vi "Dashboard Main.vi"() -> ()   [LabVIEW 2017]
uses:
  Config Cluster.ctl
  Plate Assignments.ctl
  <vilib>/Utility/miscctls.llb/LVRowAndColumnTypeDef.ctl
  <vilib>/event_ctls.llb/eventvkey.ctl
  <vilib>/Rock Robotics/Network Tables/NT Read Numeric Array.vi
  <vilib>/Rock Robotics/Network Tables/NT Read Boolean.vi
  <vilib>/Utility/file.llb/Read Delimited Spreadsheet (DBL).vi
  <vilib>/Rock Robotics/Network Tables/NT Read Boolean Array.vi
  <vilib>/Rock Robotics/Network Tables/NT Write Boolean Array.vi
  <vilib>/Rock Robotics/Network Tables/NT Write Boolean.vi
  <vilib>/Rock Robotics/Network Tables/NT Write Numeric Array.vi
  <vilib>/Utility/file.llb/Write Delimited Spreadsheet (DBL).vi
  <vilib>/Rock Robotics/WPI/Dashboard/WPI_DashboardLogging Global.vi
  <vilib>/Utility/file.llb/Read Delimited Spreadsheet (string).vi
  <vilib>/Utility/file.llb/Write Delimited Spreadsheet (string).vi
  <vilib>/Rock Robotics/Network Tables/NT Write String Array.vi
panel:
  in  "Camera Settings Right":T1={"Frame Rate"=30, "Compression"=30, "Size"=1, "DB Camera Config"=FALSE} {"Frame Rate" scale=1.0..30.0; "Compression" scale=100.0..-1.0; "Size" items=["640x480", "320x240", "160x120"]}
  in  "Camera Name Right":string(combo)="No Camera Selection"
  out "Camera Info":cluster{"Mbps LED":bool, "Mbps":dbl, "fps":dbl} {"fps" format="%#.1g"; "Mbps" format="%#.1g"}
  in  "Camera Settings":T1={"Frame Rate"=30, "Compression"=30, "Size"=1, "DB Camera Config"=FALSE} {"Frame Rate" scale=1.0..30.0; "Compression" scale=100.0..-1.0; "Size" items=["640x480", "320x240", "160x120"]}
  in  "TCP":refnum<k5>
  in  "Rec Mode":enum32{"Stop", "Record", "Playback"}(radio)
  out "Robot IP":string
  out "Image Message":string="Timeout in Camera Communications"
  in  "Dashboard Tab":T2(tab)=enum."Drive"
  out "Auto Frame":dbl
  out "Gyro":dbl
  out "Current Lift Position 2":dbl
  out "Lift Reference Point 2":dbl
  out "Zero Feedback":bool
  in  "Reset Lift to Start Config":bool
  in  "Zero Gyro":bool
  out "Flush feedback":bool
  in  "Flush Network Table":bool
  in  "Invert Manual Lift":bool
  out "Pause Cycling":bool
  in  "Config Cluster File Path":path=path "C:/Users/PhyXTGears/Desktop/ConfigCSV - 2018.csv"
  in  "Auto Array File Path":path=path "C:/Users/PhyXTGears/Desktop/AutoCSV - 2018.csv"
  out "Alt Numeric Process":dbl
  out "Alt Process Variable":bool
  in  "Select Auto":string(combo)="Select Autonomous ..."
  out "NT Connection":bool
  out "JS1 Z":dbl(slide) scale=-1.0..1.0 scale format="%#_2e"
  out "JS1 Graph":cluster{"X":dbl, "Y":dbl}[](graph)
  out "JS1 Buttons":T3
  out "JS2 Z":dbl(slide) scale=-1.0..1.0 scale format="%#_2e"
  out "JS2 Graph":cluster{"X":dbl, "Y":dbl}[](graph)
  out "JS2 Buttons":T3
  out "Mode":T4(ring)=enum."Auto Disabled"
  out "Camera Image Right":T5(plugin-control)
  out "Plate Assignments":T6
  out "Lift Reference Point":dbl
  out "Ramp Tail Status":bool=TRUE
  out "Intake Short":bool
  out "Intake Long":bool
  out "Drive Orientation":bool
  out "Current Lift Position":dbl
  out "BR Spin":dbl(knob) scale=0.0..360.0
  out "BL Spin":dbl(knob) scale=0.0..360.0
  out "FR Spin":dbl(knob) scale=0.0..360.0
  out "FL Spin":dbl(knob) scale=0.0..360.0
  out "Cube Secured":bool
  out "Cube Seen":bool
  out "Gyro":dbl(knob) scale=-180.0..180.0
  out "Lift Position":dbl(slide) scale=0.0..240000.0
  out "Time Remaining":dbl=135.0 format="%#.0f"
  out "Auto Indicator":string="Error - Driver Station Not Running"
  in  "Auto Select":string(combo)="Drive Forward"
  out "Notify LED":bool
  out "Notify":string="Error - DS Not Running"
  out "Auto Ready":bool
  out "# of Cells\nPresent":dbl
  out "Feedback":bool
  in  "Write to Sheet":bool
  in  "Arm Write":bool
  in  "Arm Read":bool
  in  "Read Sheet":bool
  in  "Auto Array":string[][](array[string])=[["", ""], ["", ""], ["", ""], ["", ""], ["", ""], ["", ""], ["", ""], ["", ""], ["", ""], ["", ""], ["", ""], ["", ""], ["", ""], ["", ""], ["", ""], ["", ""], ["", ""], ["", ""], ["", ""], ["", ""], ["", ""], ["", ""], ["", ""], ["", ""], ["", ""], ["", ""], ["", ""], ["", ""]]
  out "Auto Array 2":string[][](array[string])
  in  "Arm Write Config":bool
  in  "Config Cluster":T7
  in  "Arm Read Config":bool
  in  "Write to Sheet 2":bool
  out "Feedback 2":bool
  in  "Read Sheet 2":bool
  out "Control Feedback":bool
  in  "Zero BR":bool
  in  "Zero BL":bool
  in  "Zero FR":bool
  in  "Zero FL":bool
  out "BL Rverse":bool
  out "FL Rverse":bool
  out "BR Rverse":bool
  out "FR Rverse":bool
  in  "Enable Zero Ctrls":bool
  in  "Read Zeros from File":bool
  in  "Save Zeros to File":bool
  in  "Zero Drive":bool
  out "FR Encoder":dbl
  out "Swerve Zeros":dbl[](array[numeric])
  out "BR Spin":dbl
  out "BL Spin":dbl
  out "FR Spin":dbl
  out "FL Spin":dbl
  out "Spin Wheels":cluster{dbl, dbl, dbl, dbl}(knob) scale=0.0..360.0
  in  "Test Slider":dbl(slide) scale=0.0..100.0 scale format="%#_3g"
  in  "On/Off":bool caption="Solenoid"
  in  "Test Name":u16(ring) items=["Select the test to run..."]
  in  "Test Tree":string(tree)
  in  "Motor":cluster{"Value":dbl, "Enable":bool} {"Value" scale=-1.0..1.0 scale format="%#_3g"}
  out "Progress":T8 {"Test Progress" scale=0.0..100.0}
  in  "Rev/Fwd":cluster{"Forward":bool, "Reverse":bool}
  in  "Test Ring":u16(ring) items=["Monochrome", "Color"]
  out "Cmd Status":string
  in  "Execute Command":bool
  in  "Command Params":string[][](table)
  in  "Command Selection":i32(listbox)
  in  "CheckList":i32(listbox)
  out "Tree":string(tree)
  out "Camera Image":T5(plugin-control)
  out "Background":bool
  in  "Camera Name":string(combo)="No Camera Selection"
  # "HW"
  # "HW"
  # "Joysticks"
  # "Auto Commands Ref\nS - Stop/Abort\nT - Movement Angle\nM - Distance to move\nA -  Angle to face\nL - Lift Position"
  # "Oppo"
  # "Scale"
  # "Ours"
  # "See\nBackend\ntab for \ncmd refs"
  # "Intake"
  # "Servos"
  # "FL-Red\nFR-Orng\nBL-Grn\nBR-Blu"
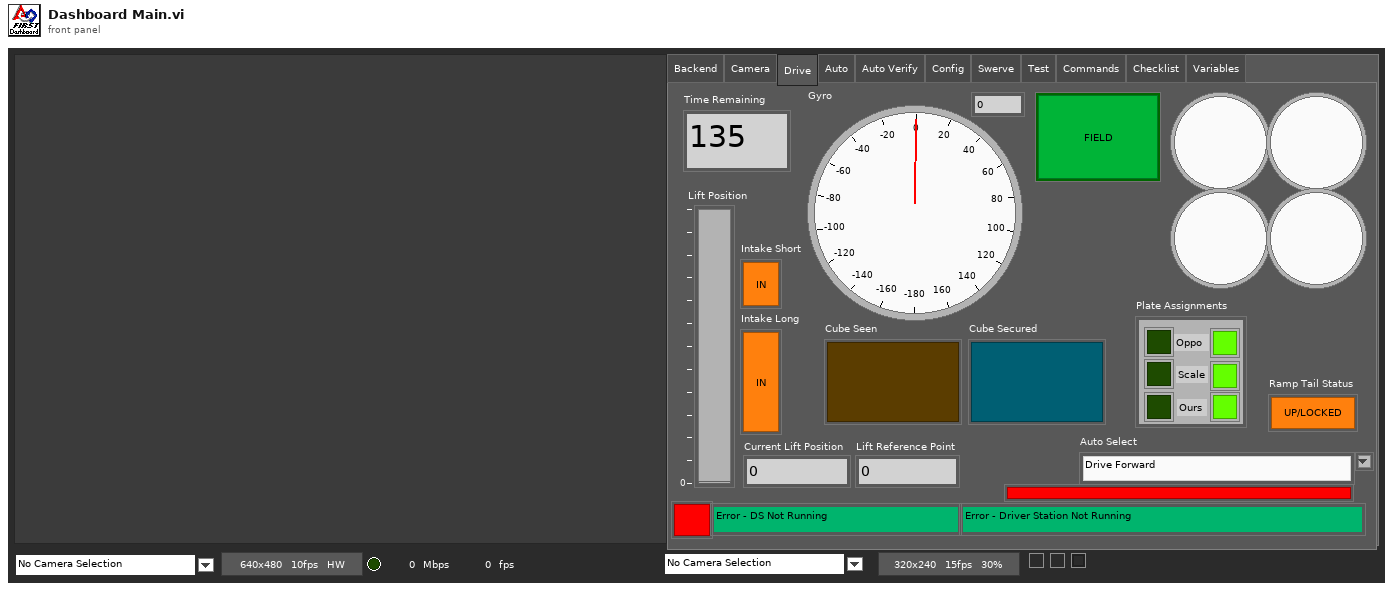
[diagram p1: front panel]
types:
  T1 = cluster{"Frame Rate":i32, "Compression":i32, "Size":u16, "DB Camera Config":bool}
  T2 = enum32{"Backend", "Camera", "Drive", "Auto", "Auto Verify", "Config", "Swerve", "Test", "Commands", "Checklist", "Variables"}
  T3 = cluster{bool, bool, bool, bool, bool, bool, bool, bool, bool, bool, bool, bool}
  T4 = enum8{"Tele-Op Disabled", "Tele-Op Enabled", "Auto Disabled", "Auto Enabled", "Test Disabled", "Test Enabled", "Disconnected", "No Code", "E-Stop"}
  T5 = typedef "IMAQ Image.ctl" = refnum<image>
  T6 = typedef "Plate Assignments.ctl" = cluster{"L Switch":bool, "R Switch":bool, "L Scale":bool, "R Scale":bool, "L Switch Opponent":bool, "R Switch Opponent":bool}
  T7 = typedef "Config Cluster.ctl" = cluster{"Intake Position Offset":dbl, "Cube Hold Position Offset":dbl, "Switch Position Offset":dbl, "Scale Position Low Offset":dbl, "Scale Position Mid Offset":dbl, "Scale Position High Offset":dbl, "Cycle Timeout":dbl, "Cycle Pause":dbl, "Carriage Intake":dbl, "Carriage Eject":dbl, "Climb Position Offset":dbl, "Intk Wheel Intk Speed":dbl, "Ramp Release Angle L":dbl, "Ramp Hold Angle L":dbl, "Ramp Release Angle R":dbl, "Ramp Hold Angle R":dbl, "Deploy Hook Angle":dbl, "Hold Hook Angle":dbl, "Reset Position Offset":dbl, "PreAdjust Position Offset":dbl, "Adjusted Position Offset":dbl, "Adjust Position Speed":dbl, "Take Slack Speed":dbl, "Carriage Slow Eject":dbl}
  T8 = cluster{"Test Progress":u8, "Test Progress Text":string}
  T9 = cluster{"Save Path":path, "Interval (s)":dbl, "Keep":i32}
  T10 = enum32{"Drive", "Camera", "Basic", "Custom", "Test", "Commands", "Checklist", "Variables"}
  T11 = typedef "Image Type" = u32
  T12 = cluster{"IDs":cluster{"RPC field ID":u16, "Unique ID":u16}, "String":string}
  T13 = cluster{"first row[0]":dbl, "first row[1]":dbl, "first row[2]":dbl, "first row[3]":dbl, "first row[4]":dbl, "first row[5]":dbl, "first row[6]":dbl, "first row[7]":dbl, "first row[8]":dbl, "first row[9]":dbl, "first row[10]":dbl, "first row[11]":dbl, "first row[12]":dbl, "first row[13]":dbl, "first row[14]":dbl, "first row[15]":dbl, "first row[16]":dbl, "first row[17]":dbl, "first row[18]":dbl, "first row[19]":dbl, "first row[20]":dbl, "first row[21]":dbl, "first row[22]":dbl, "first row[23]":dbl}
  T14 = enum8{"Enabled", "Disabled", "Disabled and Grayed Out"}
  T15 = cluster{"Error Strings":string, "Disable Counts":cluster{u16, u16}, "Rail Faults":cluster{u16, u16, u16}, "Robot IP":string, "DB Mode":u8, "Event Info":cluster{"Name":string, "Type":u8, "Number":u16, "Replay":u8}}
  T16 = cluster{"Storage":cluster{"Disk Free":u64, "RAM Block":u32, "RAM free":u32}, "CPU Utilization":cluster{"CPU % ISR":sgl, "CPU % Time Crit":sgl, "CPU % Timed Str":sgl, "CPU % High":sgl, "CPU % Above":sgl, "CPU % Normal":sgl, "CPU % Low":sgl}, "CAN":cluster{"% Bus Utilization":sgl, "Bus Off Cnt":u32, "TX_FIFO Full Cnt":u32, "Receive Error Cnt":u8, "Transmit Error Cnt":u8}, "HID":cluster{"HID Outputs":u32, "Rumble Low":u16, "Rumble High":u16}[]}
  T17 = cluster{"Status bits":cluster{"Test Mode":bool, "Autonomous":bool, "Enabled":bool, "Code Start":bool, "Brownout":bool, "Reserved 2":bool, "Reserved 3":bool, "E-Stop":bool}, "Code Trace":cluster{"Disabled":bool, "TeleOp":bool, "Auto":bool, "Test":bool}, "Controller Type":enum16{"unknown", "cRIO", "roboRio"}, "Code?":enum16{"unknown", "noCode", "code"}, "Battery V":dbl}
  T18 = cluster{"Control Bits":cluster{"TestMode":bool, "Autonomous":bool, "Enabled":bool, "FMS Present":bool, bool, bool, bool, "E-Stop":bool}, "Team Station ":u8, "Countdown":sgl, "Joystick Values":cluster{"Axes":dbl[], "Buttons":bool[], "POVs":i16[]}[]}
  T19 = cluster{"Axes":dbl[], "Buttons":bool[], "POVs":i16[]}[]
  T20 = cluster{"Axes":dbl[], "Buttons":bool[], "POVs":i16[]}
  T21 = cluster{"Buttons[0]":bool, "Buttons[1]":bool, "Buttons[2]":bool, "Buttons[3]":bool, "Buttons[4]":bool, "Buttons[5]":bool, "Buttons[6]":bool, "Buttons[7]":bool, "Buttons[8]":bool, "Buttons[9]":bool, "Buttons[10]":bool, "Buttons[11]":bool}
  T22 = cluster{"Angle":dbl, "Angle":dbl, "Angle":dbl, "Angle":dbl}
  T23 = cluster{"Camera Image":refnum<vi>, "Dashboard Tab":refnum<vi>, "Background":refnum<vi>, "Rec Mode":refnum<vi>, "Test Slider":refnum<vi>, "On/Off ":refnum<vi>, "Test Ring":refnum<vi>, "Rev/Fwd":refnum<vi>, "Test Name":refnum<vi>, "Motor":refnum<vi>, "Progress":refnum<vi>, "CheckList":refnum<vi>, "Tree":refnum<vi>, "Test Tree":refnum<vi>, "Command Params":refnum<vi>, "Command Selection":refnum<vi>, "Execute Command":refnum<vi>, "Cmd Status":refnum<vi>, "Camera Settings":refnum<vi>, "Camera Name":refnum<vi>, "Camera Info":refnum<vi>, "Camera Settings Right":refnum<vi>, "Camera Name Right":refnum<vi>, "Camera Image Right":refnum<vi>}
  T24 = cluster{"Camera Name":string, string, "Saved DB Images Info":cluster{"Save Path":path, "Interval (s)":dbl, "Keep":i32}}
  T25 = cluster{"Camera Name Right":string, string, "Saved DB Images Info":cluster{"Save Path":path, "Interval (s)":dbl, "Keep":i32}}
  T26 = cluster{"Operation":enum16{"Update", "Clear"}, "Color Box":u32}[]
  T27 = typedef "eventvkey.ctl" = enum16{"ASCII", "Enter", "Return", "Shift", "Ctrl", "Alt", "Cmd", "Opt", "Caps", "NumLock", "Clear", "Break", "Up", "Down", "Left", "Right", "Insert", "Delete", "Home", "End", "PageUp", "PageDown", "Escape", "Help", "Pause", "ScrollLock", "F1", "F2", "F3", "F4", "F5", "F6", "F7", "F8", "F9", "F10", "F11", "F12", "F13", "F14", "F15", "F16", "F17", "F18", "F19", "F20", "F21", "F22", "F23", "F24", "Play", "VolumeUp", "VolumeDown", "Mute", "Two Byte Char"}
  T28 = cluster{"Image Size":bool, "Image Type":bool, "Pixel Value":bool, "ROI Information":bool, "Zoom Factor":bool}
  T29 = cluster{"Operation":enum16{"Update", "Clear"}, "Color Box":u32}
  T30 = typedef "LVRowAndColumnTypeDef.ctl" = cluster{"Row":i32, "Column":i32}
  T31 = cluster{"Shift":bool, "Ctrl":bool, "Alt":bool, "Cmd":bool, "Opt":bool}
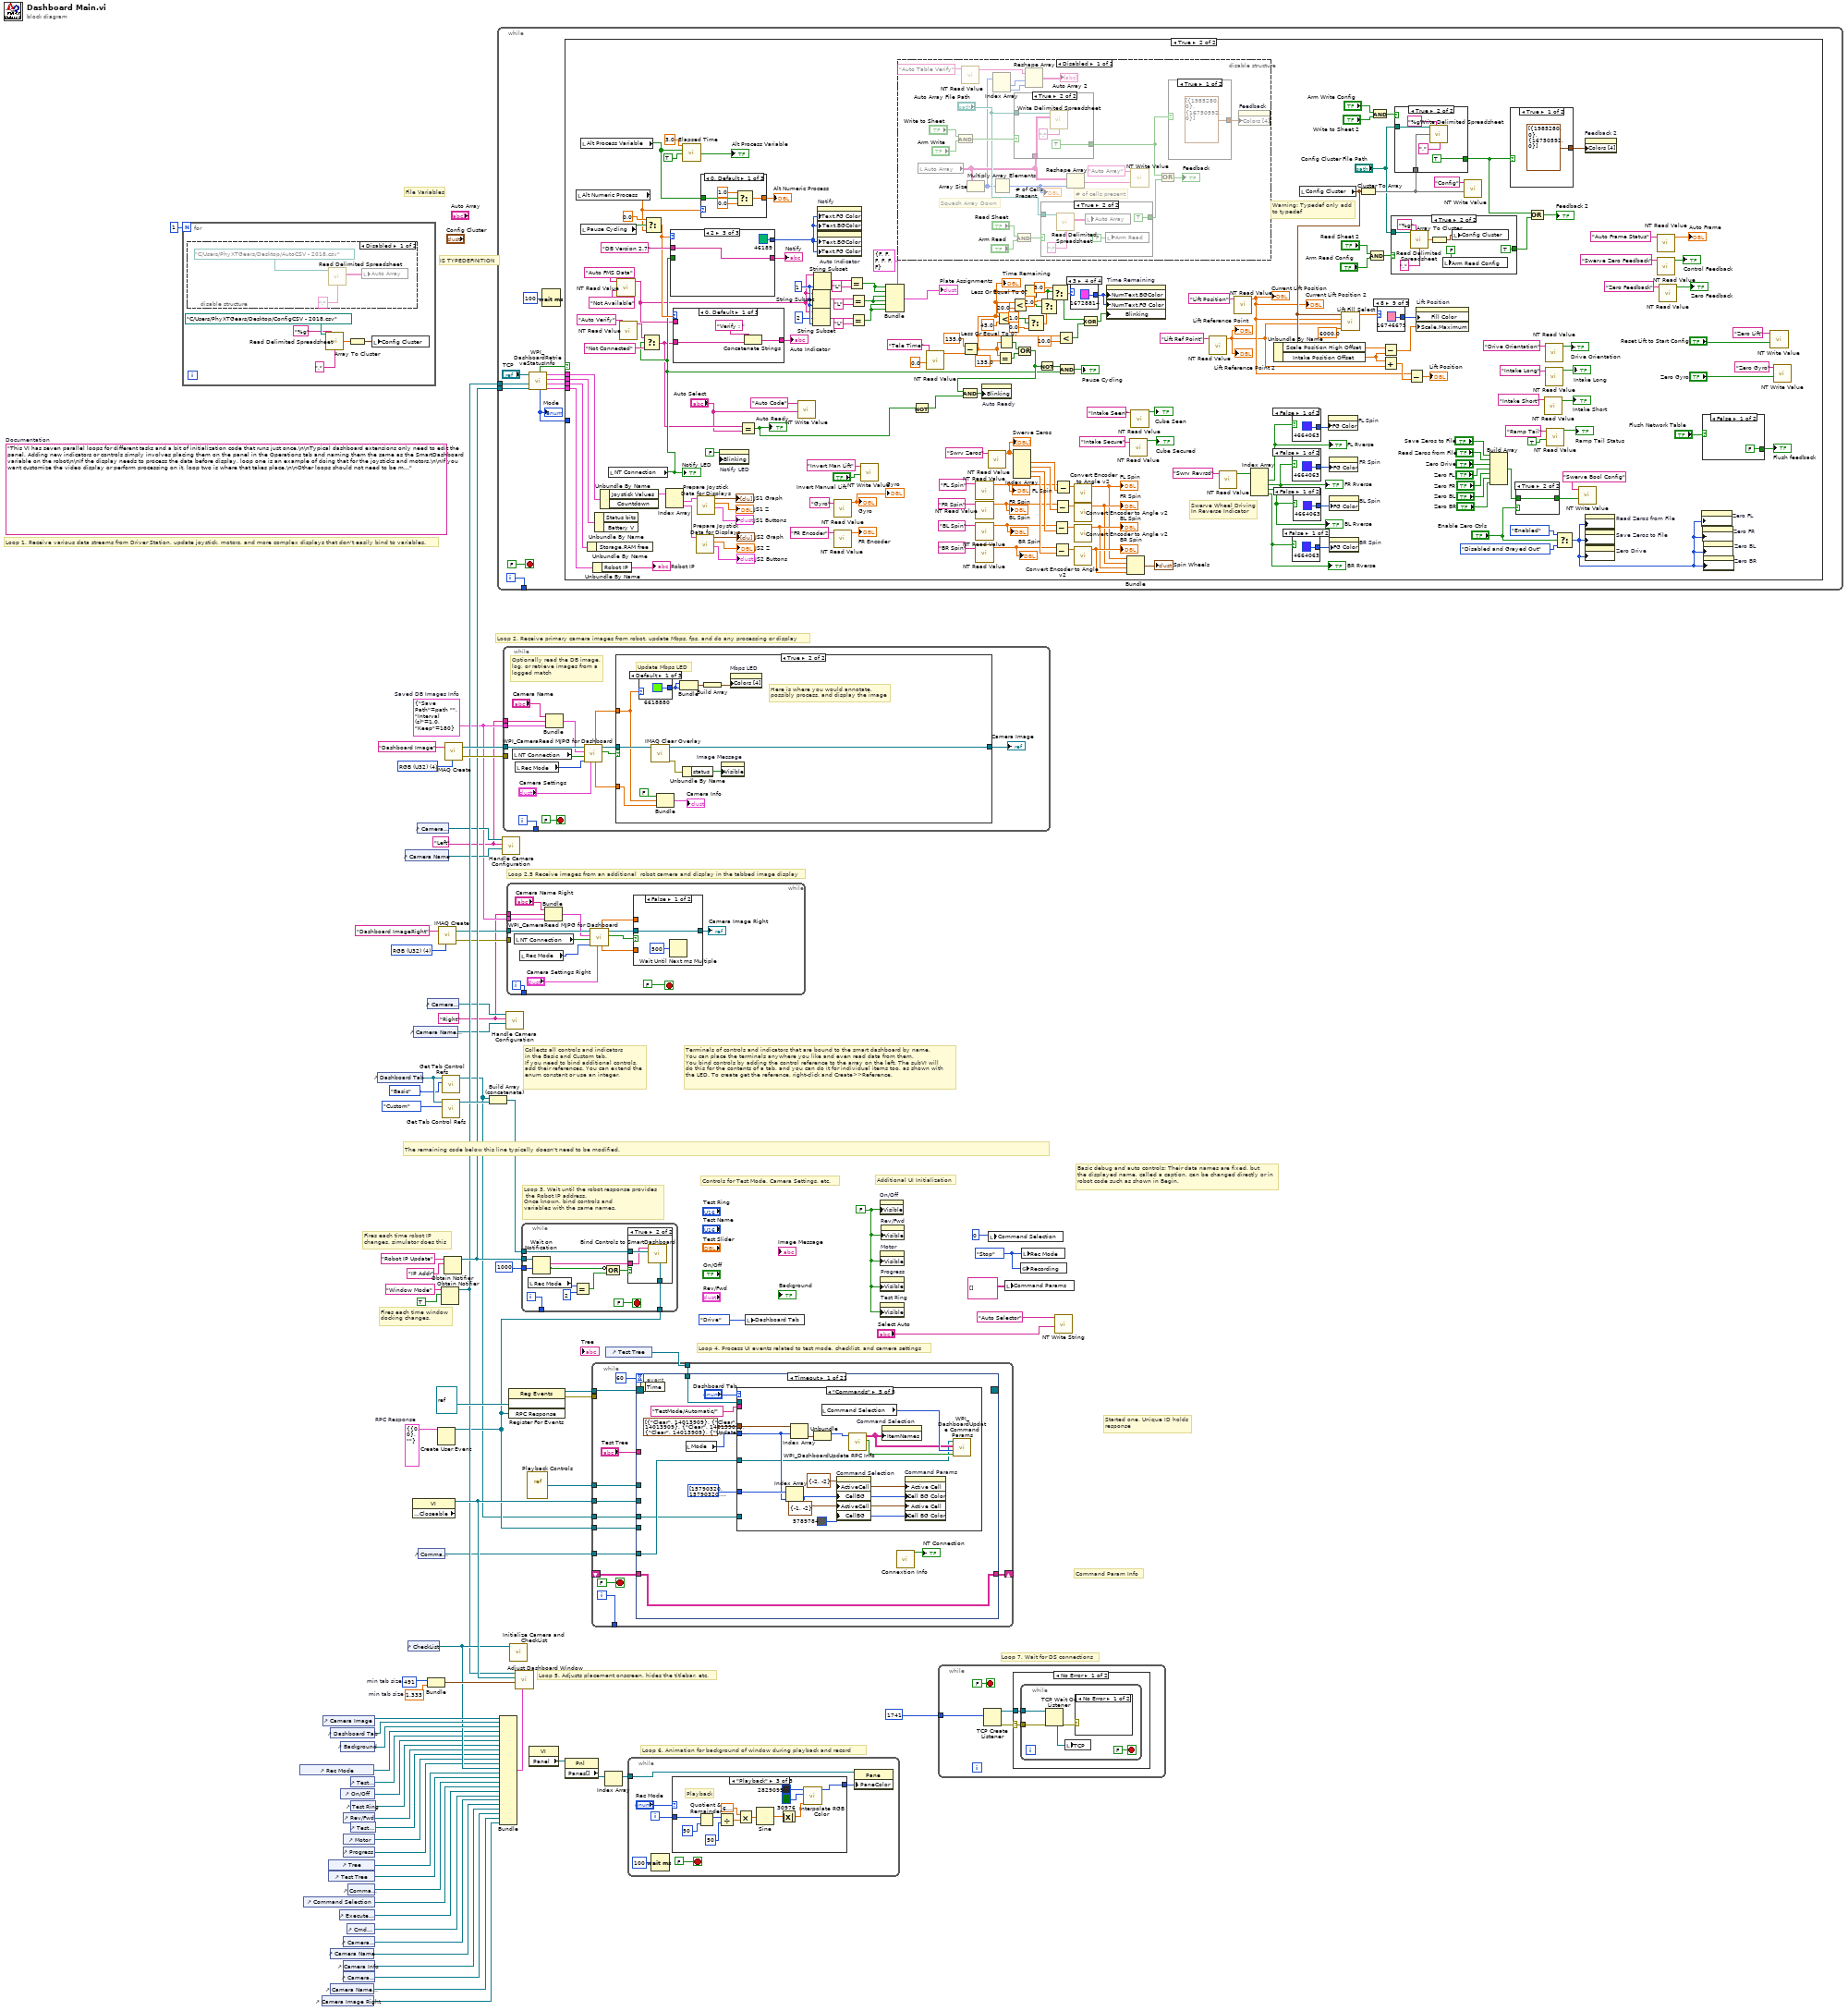
[diagram p0: block diagram]
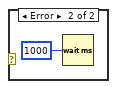
[diagram p4: hidden frame]
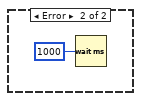
[diagram p5: hidden frame]
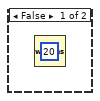
[diagram p6: hidden frame]
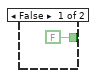
[diagram p7: hidden frame]
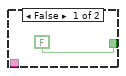
[diagram p8: hidden frame]
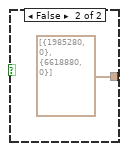
[diagram p9: hidden frame]
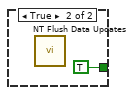
[diagram p11: hidden frame]
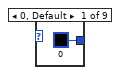
[diagram p12: hidden frame]
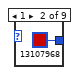
[diagram p13: hidden frame]
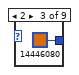
[diagram p14: hidden frame]
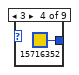
[diagram p15: hidden frame]
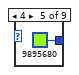
[diagram p16: hidden frame]
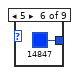
[diagram p17: hidden frame]
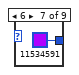
[diagram p18: hidden frame]
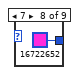
[diagram p19: hidden frame]
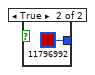
[diagram p20: hidden frame]
diagram:
  w4 = T9 {"Save Path"=path "", "Interval (s)"=1.0, "Keep"=180}  # Saved DB Images Info
  w3 = "Right"
  w2 = "Left"
  w14 = T11 4 items=["Grayscale (U8)", "Grayscale (I16)", "Grayscale (SGL)", "Complex (CSG)", "RGB (U32)", "HSL (U32)", "RGB (U64)"] ("Image Type")
  w30 = T12 {"IDs"={"RPC field ID"=0, "Unique ID"=0}, "String"=""}  # RPC Response
  w53 = 491  # min tab size
  w52 = 1.333  # min tab size
  w60 = enum32{"Stop", "Record", "Playback"}."Stop" ("Rec Mode")
  w37 = FALSE ("Visible")
  (unwired) "This VI has seven parallel loops for different tasks and a bit of initialization code that runs just once.\n\nTypical dashboard extensions only need to edit the panel. Adding new indicators or controls simply involves placing them on the panel in the Operations tab and naming them the same as the SmartDashboard variable on the robot\n\nIf the display needs to process the data before display, loop one is an example of doing that for the joysticks and motors.\n\nIf you want customize the video display or perform processing on it, loop two is where that takes place.\n\nOther loops should not need to be modified. They are pretty standard, and document the task they perform."  # Documentation
  w77 = T11 4 items=["Grayscale (U8)", "Grayscale (I16)", "Grayscale (SGL)", "Complex (CSG)", "RGB (U32)", "HSL (U32)", "RGB (U64)"] ("Image Type")
  # "IS TYPEDEFINITION"
  # "File Variables"
  # "Loop 2.5 Receive images from an additional  robot camera and display in the tabbed image display"
  # "Command Param Info"
  # "Started one, Unique ID holds\nresponse"
  # "Loop 7. Wait for DS connections"
  # "Basic debug and auto controls: Their data names are fixed, but\nthe displayed name, called a caption, can be changed directly or in\nrobot code such as shown in Begin."
  # "Controls for Test Mode, Camera Settings, etc."
  # "Additional UI Initialization"
  # "Loop 6. Animation for background of window during playback and record"
  # "Fires each time robot IP\nchanges, simulator does this"
  # "Fires each time window\ndocking changes."
  # "Collects all controls and indicators\nin the Basic and Custom tab.\nIf you need to bind additional controls,\nadd their references. You can extend the\nenum constant or use an integer."
  # "The remaining code below this line typically doesn't need to be modified."
  # "Loop 4. Process UI events related to test mode, checklist, and camera settings"
  # "Terminals of controls and indicators that are bound to the smart dashboard by name.\nYou can place the terminals anywhere you like and even read data from them.\nYou bind controls by adding the control reference to the array on the left. The subVI will\ndo this for the contents of a tab, and you can do it for individual items too, as shown with\nthe LED. To create get the reference, right-click and Create>>Reference."
  # "Loop 3. Wait until the robot response provides\n the Robot IP address.\nOnce known, bind controls and\nvariables with the same names."
  # "Loop 5. Adjusts placement onscreen, hides the titlebar, etc."
  # "Loop 1. Receive various data streams from Driver Station, update joystick, motors, and more complex displays that don't easily bind to variables."
  # "Loop 2. Receive primary camera images from robot, update Mbps, fps, and do any processing or display"
  n1 = for {
    N: 1 -> [_]
    n2 = disable-structure shown="Disabled" {
      frame Disabled {
        n3 = call-poly <vilib>:"Read Delimited Spreadsheet.vi"("file path (dialog if empty)"=path "C:/Users/PhyXTGears/Desktop/AutoCSV - 2018.csv", "delimiter (\\t)"=":" ("delimiter (\\t)")) -> ("all rows"=w84:string[][])  [unwired: 8 in, 5 out]
        n4 = local write "Auto Array"(w84) -> ()
      }
      frame Enabled {
      }
    }
    n5 = call-poly <vilib>:"Read Delimited Spreadsheet.vi"("file path (dialog if empty)"=path "C:/Users/PhyXTGears/Desktop/ConfigCSV - 2018.csv", "format (%.3f)"="%g", "delimiter (\\t)"="," ("delimiter (\\t)")) -> ("first row"=w79:dbl[])  [unwired: 7 in, 5 out]
    n6 = Array To Cluster(array=w79) -> (cluster=w78:T13)
    n7 = local write "Config Cluster"(w78) -> ()
  }
  n8 = control-ref of="Rec Mode"() -> (w43:refnum<vi>)
  n9 = control-ref of="Command Selection"() -> (w29:refnum<vi>)
  n10 = control-ref of="Camera Image Right"() -> (w7:refnum<vi>)
  n11 = control-ref of="Camera Image"() -> (w55:refnum<vi>)
  n12 = control-ref of="Tree"() -> (w47:refnum<vi>)
  n13 = control-ref of="Test Tree"() -> (w46:refnum<vi>)
  n14 = control-ref of="Dashboard Tab"() -> (w54:refnum<vi>)
  n15 = control-ref of="Camera Name"() -> (w20:refnum<vi>)
  n16 = control-ref of="Camera Name Right"() -> (w8:refnum<vi>)
  n17 = control-ref of="Execute Command"() -> (w31:refnum<vi>)
  n18 = control-ref of="Background"() -> (w50:refnum<vi>)
  n19 = control-ref of="On/Off"() -> (w41:refnum<vi>)
  n20 = control-ref of="Progress"() -> (w38:refnum<vi>)
  n21 = control-ref of="Camera Settings"() -> (w21:refnum<vi>)
  n22 = control-ref of="Camera Info"() -> (w19:refnum<vi>)
  n23 = control-ref of="Camera Settings Right"() -> (w9:refnum<vi>)
  n24 = control-ref of="Rev/Fwd"() -> (w39:refnum<vi>)
  n25 = control-ref of="Motor"() -> (w44:refnum<vi>)
  n26 = control-ref of="Cmd Status"() -> (w25:refnum<vi>)
  n27 = control-ref of="Command Params"() -> (w32:refnum<vi>)
  n28 = control-ref of="Test Slider"() -> (w42:refnum<vi>)
  n29 = control-ref of="Test Ring"() -> (w40:refnum<vi>)
  n30 = control-ref of="Test Name"() -> (w45:refnum<vi>)
  n31 = control-ref of="Dashboard Tab"() -> (w58:refnum<vi>)
  n32 = control-ref of="Camera Name"() -> (w22:refnum<vi>)
  n33 = control-ref of="CheckList"() -> (w48:refnum<vi>)
  n34 = property class="VI" props=["Front Panel.Closeable"]() -> (reference out=w59:refnum<vi>)  [unwired: 2 in, 2 out]
  n35 = control-ref of="Camera Name Right"() -> (w10:refnum<vi>)
  n36 = control-ref of="Camera Settings"() -> (w23:refnum<vi>)
  n37 = control-ref of="Command Params"() -> (w24:refnum<vi>)
  n38 = control-ref of="Camera Settings Right"() -> (w11:refnum<vi>)
  n39 = Bundle("min tab size"=w53, "min tab size"=w52) -> (w51:cluster{"min tab size":i32, "min tab size":dbl})  [unwired: 1 in]
  n40 = Create User Event(user event datatype=w30) -> (user event=w26:refnum<user-event>)  [unwired: 1 in, 1 out]
  n41 = call "IMAQ Create"("Image Name"="Dashboard ImageRight", "Image Type"=w14) -> ("New Image"=w13:T5, "error out"=w12:errorcluster)  [unwired: 2 in, 1 out]
  n42 = Obtain Notifier(name (unnamed)="Window Mode", notification data type=TRUE) -> (notifier out=w35:refnum<notifier>)  [unwired: 2 in, 2 out]
  n43 = call <vilib>:"Get Tab Control Refs.vi"("Page Index"=T10."Basic" ("Dashboard Tab"), "TabControl in"=w58) -> ("ControlsOnPage"=w18:refnum<vi>[])  [unwired: 9 in]
  n44 = call <vilib>:"Get Tab Control Refs.vi"("Page Index"=T10."Custom" ("Dashboard Tab"), "TabControl in"=w58) -> ("ControlsOnPage"=w57:refnum<vi>[])  [unwired: 9 in]
  n45 = Obtain Notifier(name (unnamed)="Robot IP Update", notification data type="IP Addr" ("name (unnamed)")) -> (notifier out=w36:refnum<notifier>)  [unwired: 2 in, 2 out]
  n46 = call "IMAQ Create"("Image Name"="Dashboard Image", "Image Type"=w77) -> ("New Image"=w75:T5, "error out"=w74:errorcluster)  [unwired: 2 in, 1 out]
  n47 = Build Array (concatenate)(w18, w57) -> (w56:refnum<vi>[])
  n48 = while {
    tunnel: [w96] -> _
    tunnel: w36 -> [w90]
    tunnel: w35 -> [w87]
    i -> [w96]
    stop <- FALSE stop-if-true
    n49 = call <vilib>:"WPI_DashboardRetrieveStatusInfo.vi"("Binding Refnum"=w90, "Window Mode Notifier"=w87, "TCP Cnx"="TCP") -> ("Power and Errors"=w91:T15, "Robot Metrics"=w94:T16, "Status Info"=w95:T17, "Control Info"=w92:T18, "Robot Mode"=w89:T4, "Process?"=w93:bool)  [unwired: 3 in]
    "Mode" <- w89
    n50 = Wait (ms)(milliseconds to wait=u32 100) -> ()  [unwired: 1 out]
    n51 = case shown="True" w93 {
      tunnel: w95 -> [_ w283]
      tunnel: w94 -> [_ w282]
      tunnel: w92 -> [_ w281]
      tunnel: w91 -> [_ w280]
      tunnel: w89 -> [_ _]
      frame False {
        n52 = Wait (ms)(milliseconds to wait=u32 20) -> ()  [unwired: 1 out]
      }
      frame True {
        w137 = 1 ("length (rest)")
        # "Swerve Wheel Driving\nIn Reverse Indicator"
        # "Warning: Typedef only add\nto typedef"
        n53 = local read "Alt Numeric Process"() -> (w236:dbl)
        n54 = local read "Pause Cycling"() -> (w237:bool)
        n55 = local read "Alt Process Variable"() -> (w267:bool)
        n56 = Unbundle By Name(w282) -> ()  [unwired: 1 out]
        n57 = Unbundle By Name(w280) -> ("Robot IP"=→"Robot IP":string)
        n58 = Unbundle By Name(w283) -> ()  [unwired: 2 out]
        n59 = Unbundle By Name(w281) -> ("Joystick Values"=w279:T19)  [unwired: 1 out]
        n60 = local read "NT Connection"() -> (w234:bool)
        "Notify LED" <- w234
        n61 = call-poly <vilib>:"NT Read Value.vi"("Default Value"="Not Available", "Name"="Auto FMS Data") -> ("String"=w135:string)  [unwired: 8 in, 1 out]
        n62 = call-poly <vilib>:"NT Read Value.vi"("Name"="Auto Verify") -> ("String"=w243:string)  [unwired: 9 in, 1 out]
        n63 = Select(t=w243, s=w234, f="Not Connected") -> (s? t:f=w233:string)
        n64 = Select(t=0.0, s=w237, f=w236) -> (s? t:f=w235:dbl)
        n65 = Index Array(array=w279) -> (element #1=w278:T20, element #2=w274:T20)  [unwired: 2 in]
        n66 = case shown="2" w235 {
          tunnel: [w372 w379 w382] -> w264
          tunnel: w234 -> [w374 _ _]
          tunnel: "DB Version 2.7" ("Notify") -> [_ _ w382]
          tunnel: [u32 13816530 u32 8898560 u32 46189] -> w209
          frame 0, Default {
            n67 = Select(t="NT Connected", s=w374, f="NT Disconneted" ("Notify")) -> (s? t:f=w372:string)
          }
          frame 1 {
            n68 = call-poly <vilib>:"NT Read Value.vi"("Default Value"="No Data", "Name"="Code Version") -> ("String"=w377:string)  [unwired: 8 in, 1 out]
            n69 = Concatenate Strings("Code : " ("Default Value"), w377) -> (w379:string)
          }
          frame 2 {
          }
        }
        "Notify" <- w264
        n70 = case shown="0, Default" w235 {
          tunnel: [w356 w359 w362] -> w242
          tunnel: w233 -> [w355 _ _]
          tunnel: w135 -> [_ w358 _]
          frame 0, Default {
            n71 = Concatenate Strings("Verify : " ("Default Value"), w355) -> (w356:string)
          }
          frame 1 {
            n72 = Concatenate Strings("FMS Auto Code : " ("Default Value"), w358) -> (w359:string)
          }
          frame 2 {
            n73 = call-poly <vilib>:"NT Read Value.vi"("Default Value"="Not Available", "Name"="Auto Ran") -> ("String"=w361:string)  [unwired: 8 in, 1 out]
            n74 = Concatenate Strings("Auto Ran : " ("Default Value"), w361) -> (w362:string)
          }
        }
        "Auto Indicator" <- w242
        n75 = call "Elapsed Time"("Time Target (s)"=3.0, "Reset"=w267, "Auto Reset"=TRUE) -> ("Time has Elapsed"=→"Alt Process Variable":bool)  [unwired: 9 in, 7 out]
        n76 = call "Prepare Joystick Data for Displays.vi"("Joystick Values"=w274) -> ("Buttons"=→"JS2 Buttons":T21, "Z Axis"=→"JS2 Z":dbl, "Cartesian Data"=→"JS2 Graph":cluster{"X axis":dbl, "X axis":dbl}[])  [unwired: 8 in]
        n77 = call "Prepare Joystick Data for Displays.vi"("Joystick Values"=w278) -> ("Buttons"=→"JS1 Buttons":T21, "Z Axis"=→"JS1 Z":dbl, "Cartesian Data"=→"JS1 Graph":cluster{"X axis":dbl, "X axis":dbl}[])  [unwired: 8 in]
        n78 = case shown="0, Default" w236 {
          tunnel: w267 -> [w386 w390 w394]
          tunnel: [w383 w387 w391] -> w266
          frame 0, Default {
            n79 = Select(t=1.0, s=w386, f=0.0) -> (s? t:f=w383:dbl)
          }
          frame 1 {
            n80 = Select(t=2.0, s=w390, f=1.0) -> (s? t:f=w387:dbl)
          }
          frame 2 {
            n81 = Select(t=0.0, s=w394, f=2.0) -> (s? t:f=w391:dbl)
          }
        }
        "Alt Numeric Process" <- w266
        n82 = property on="Notify LED" class="Bool (strict)"("Blinking"=FALSE) -> ()  [unwired: 2 in, 2 out]
        n83 = Equal?(x=w233, y="Auto Select") -> (x = y?=w231:bool)
        "Auto Ready" <- w231
        n84 = call-poly <vilib>:"NT Write Value.vi"("String"="Auto Select", "Name"="Auto Code") -> ()  [unwired: 9 in, 1 out]
        n85 = String Subset(string=w135, offset (0)=w137, length (rest)=w137) -> (substring=w129:string)
        n86 = String Subset(string=w135, offset (0)=2, length (rest)=w137) -> (substring=w130:string)
        n87 = String Subset(string=w135, length (rest)=w137) -> (substring=w134:string)  [unwired: 1 in]
        n88 = property on="Notify" class="Str"("Text.FG Color"=w209, "Text.BGColor"=w209) -> ()  [unwired: 2 in, 2 out]
        n89 = property on="Auto Indicator" class="Str"("Text.BGColor"=w209, "Text.FG Color"=w209) -> ()  [unwired: 2 in, 2 out]
        n90 = call-poly <vilib>:"NT Read Value.vi"("Name"="FR Encoder" ("refnum name")) -> ("Numeric"=→"FR Encoder":dbl)  [unwired: 9 in, 1 out]
        n91 = call-poly <vilib>:"NT Read Value.vi"("Name"="Gyro" ("refnum name")) -> ("Numeric"=→"Gyro" →"Gyro":dbl)  [unwired: 9 in, 1 out]
        n92 = Equal?(x=w134, y="L") -> (x = y?=w126:bool)
        n93 = Equal?(x=w129, y="L") -> (x = y?=w125:bool)
        n94 = Equal?(x=w130, y="L") -> (x = y?=w124:bool)
        n95 = call-poly <vilib>:"NT Write Value.vi"("Boolean"="Invert Manual Lift", "Name"="Invert Man Lift") -> ()  [unwired: 9 in, 1 out]
        n96 = Bundle(cluster=T6 {"L Switch"=FALSE, "R Switch"=FALSE, "L Scale"=FALSE, "R Scale"=FALSE, "L Switch Opponent"=FALSE, "R Switch Opponent"=FALSE} ("Plate Assignments"), "L Switch"=w126, "R Switch"=w126, "L Scale"=w125, "R Scale"=w125, "L Switch Opponent"=w124, "R Switch Opponent"=w124) -> (→"Plate Assignments":T6)
        n97 = disable-structure shown="Disabled" {
          frame Disabled {
            # "Squash Array Down"
            # "# of cells present"
            n98 = local read "Auto Array"() -> (w292:string[][])
            n99 = And(x="Write to Sheet", y="Arm Write") -> (x .and. y?=w303:bool)
            n100 = call-poly <vilib>:"NT Read Value.vi"("Name"="Auto Table Verify") -> ("String Array"=w289:string[])  [unwired: 9 in, 1 out]
            n101 = Array Size(array=w292) -> (size(s)=w288:i32[])
            n102 = Index Array(array=w288) -> (element #1=w287:i32, element #2=w286:i32)  [unwired: 2 in]
            n103 = Multiply Array Elements(1:w288) -> (0:w291:i32)
            "# of Cells\nPresent" <- w291
            n104 = case shown="True" w303 {
              tunnel: "Auto Array File Path" -> [_ w314]
              tunnel: w292 -> [_ w313]
              tunnel: [FALSE ("Saved to Sheet") TRUE ("Saved to Sheet")] -> w294
              frame False {
              }
              frame True {
                n105 = call-poly <vilib>:"Write Delimited Spreadsheet.vi"("file path (dialog if empty)"=w314, "2D data"=w313, "delimiter (\\t)"=":" ("delimiter (\\t)")) -> ()  [unwired: 11 in, 2 out]
              }
            }
            n106 = And(x="Read Sheet", y="Arm Read") -> (x .and. y?=w297:bool)
            n107 = Reshape Array(w289, w287, w286) -> (→"Auto Array 2":string[][])
            n108 = case shown="True" w297 {
              tunnel: "Auto Array File Path" -> [_ w309]
              tunnel: [FALSE TRUE] -> w295
              frame False {
              }
              frame True {
                n109 = call-poly <vilib>:"Read Delimited Spreadsheet.vi"("file path (dialog if empty)"=w309, "delimiter (\\t)"=":" ("delimiter (\\t)")) -> ("all rows"=w310:string[][])  [unwired: 8 in, 5 out]
                n110 = local write "Auto Array"(w310) -> ()
                n111 = local write "Arm Read"(FALSE ("Update\nDB Table")) -> ()
              }
            }
            n112 = Reshape Array(w292, w291) -> (w284:string[])
            n113 = call-poly <vilib>:"NT Write Value.vi"("String Array"=w284, "Name"="Auto Array") -> ()  [unwired: 9 in, 1 out]
            n114 = Or(x=w294, y=w295) -> (x .or. y?=→"Feedback":bool)
            n115 = case shown="True" w294 {
              tunnel: [cluster{u32, u32}[] [{1985280, 0}, {16750592, 0}] ("Colors [4]") cluster{u32, u32}[] [{1985280, 0}, {6618880, 0}] ("Colors [4]")] -> w304
              frame True {
              }
              frame False {
              }
            }
            n116 = property on="Feedback" class="Bool (strict)"("Colors [4]"=w304) -> ()  [unwired: 2 in, 2 out]
          }
          frame Enabled {
          }
        }
        n117 = Not(x=w231) -> (.not. x?=w108:bool)
        n118 = call-poly <vilib>:"NT Read Value.vi"("Default Value"=0.0, "Name"="Tele Time") -> ("Numeric"=w251:dbl)  [unwired: 8 in, 1 out]
        n119 = Subtract(x=135.0, y=w251) -> (x-y=w140:dbl)
        "Time Remaining" <- w140
        n120 = call-poly <vilib>:"NT Read Value.vi"("Name"="FL Spin" ("refnum name")) -> ("Numeric"=w213:dbl)  [unwired: 9 in, 1 out]
        "FL Spin" <- w213
        n121 = call-poly <vilib>:"NT Read Value.vi"("Name"="FR Spin" ("refnum name")) -> ("Numeric"=w214:dbl)  [unwired: 9 in, 1 out]
        "FR Spin" <- w214
        n122 = call-poly <vilib>:"NT Read Value.vi"("Name"="BL Spin" ("refnum name")) -> ("Numeric"=w215:dbl)  [unwired: 9 in, 1 out]
        "BL Spin" <- w215
        n123 = call-poly <vilib>:"NT Read Value.vi"("Name"="BR Spin" ("refnum name")) -> ("Numeric"=w216:dbl)  [unwired: 9 in, 1 out]
        "BR Spin" <- w216
        n124 = call-poly <vilib>:"NT Read Value.vi"("Name"="Swrv Zeros") -> ("Numeric Array"=w212:dbl[])  [unwired: 9 in, 1 out]
        "Swerve Zeros" <- w212
        n125 = Less?(x=w140, y=45.0) -> (x < y?=w257:bool)
        n126 = Equal?(x=w140, y=135.0) -> (x = y?=w248:bool)
        n127 = Less Or Equal To 0?(x=w140) -> (x <= 0?=w247:bool)
        n128 = Less?(x=w140, y=20.0) -> (x < y?=w142:bool)
        n129 = Index Array(array=w212) -> (element #1=w218:dbl, element #2=w219:dbl, element #3=w220:dbl, element #4=w221:dbl)  [unwired: 4 in]
        n130 = Or(x=w247, y=w248) -> (x .or. y?=w238:bool)
        n131 = And(x=w238, y=w108) -> (x .and. y?=w241:bool)
        n132 = property on="Auto Ready" class="Bool (strict)"("Blinking"=w241) -> ()  [unwired: 2 in, 2 out]
        n133 = Less Or Equal To 0?(x=w140) -> (x <= 0?=w105:bool)
        n134 = Select(t=1.0, s=w257, f=0.0) -> (s? t:f=w259:dbl)
        n135 = Not(x=w238) -> (.not. x?=w239:bool)
        n136 = Select(t=2.0, s=w142, f=w259) -> (s? t:f=w260:dbl)
        n137 = Select(t=3.0, s=w105, f=w260) -> (s? t:f=w261:dbl)
        n138 = Subtract(x=w215, y=w220) -> (x-y=w224:dbl)
        n139 = Subtract(x=w216, y=w221) -> (x-y=w223:dbl)
        n140 = Subtract(x=w214, y=w219) -> (x-y=w225:dbl)
        n141 = Subtract(x=w213, y=w218) -> (x-y=w226:dbl)
        n142 = Less?(x=w140, y=10.0) -> (x < y?=w107:bool)
        n143 = And(x=w239, y=w234) -> (x .and. y?=→"Pause Cycling":bool)
        n144 = case shown="3" w261 {
          tunnel: [u32 13816530 u32 16769536 u32 16755712 u32 16728814] -> w232
          frame 0, Default {
          }
          frame 1 {
          }
          frame 2 {
          }
          frame 3 {
          }
        }
        n145 = call "Convert Encoder to Angle v2.vi"("Encoder Units"=w226) -> ("Angle"=w176:dbl)  [unwired: 9 in, 1 out]
        "FL Spin" <- w176
        n146 = call "Convert Encoder to Angle v2.vi"("Encoder Units"=w225) -> ("Angle"=w177:dbl)  [unwired: 9 in, 1 out]
        "FR Spin" <- w177
        n147 = call "Convert Encoder to Angle v2.vi"("Encoder Units"=w224) -> ("Angle"=w178:dbl)  [unwired: 9 in, 1 out]
        "BL Spin" <- w178
        n148 = call "Convert Encoder to Angle v2.vi"("Encoder Units"=w223) -> ("Angle"=w179:dbl)  [unwired: 9 in, 1 out]
        "BR Spin" <- w179
        n149 = Exclusive Or(1:w107, 2:w105) -> (0:w106:bool)
        n150 = property on="Time Remaining" class="DigNum (strict)"("NumText.BGColor"=w232, "NumText.FG Color"=w232, "Blinking"=w106) -> ()  [unwired: 2 in, 2 out]
        n151 = Bundle("Angle"=w176, "Angle"=w177, "Angle"=w178, "Angle"=w179) -> (→"Spin Wheels":T22)  [unwired: 1 in]
        n152 = call-poly <vilib>:"NT Read Value.vi"("Name"="Intake Secure" ("refnum name")) -> ("Boolean"=→"Cube Secured":bool)  [unwired: 9 in, 1 out]
        n153 = call-poly <vilib>:"NT Read Value.vi"("Name"="Intake Seen" ("refnum name")) -> ("Boolean"=→"Cube Seen":bool)  [unwired: 9 in, 1 out]
        n154 = call-poly <vilib>:"NT Read Value.vi"("Name"="Lift Ref Point") -> ("Numeric"=w111:dbl)  [unwired: 9 in, 1 out]
        "Lift Reference Point" <- w111
        "Lift Reference Point 2" <- w111
        n155 = call-poly <vilib>:"NT Read Value.vi"("Name"="Swrv Revrsd") -> ("Boolean Array"=w180:bool[])  [unwired: 9 in, 1 out]
        n156 = call-poly <vilib>:"NT Read Value.vi"("Name"="Lift Position" ("refnum name")) -> ("Numeric"=w112:dbl)  [unwired: 9 in, 1 out]
        "Current Lift Position" <- w112
        "Current Lift Position 2" <- w112
        n157 = Index Array(array=w180) -> (element #1=w174:bool, element #2=w173:bool, element #3=w171:bool, element #4=w168:bool)  [unwired: 4 in]
        "FR Rverse" <- w173
        "BR Rverse" <- w168
        "FL Rverse" <- w174
        "BL Rverse" <- w171
        n158 = case shown="False" w168 {
          tunnel: [u32 4664063 u32 11796992] -> w169
          frame False {
          }
          frame True {
          }
        }
        n159 = case shown="False" w174 {
          tunnel: [u32 4664063 u32 11796992] -> w175
          frame False {
          }
          frame True {
          }
        }
        n160 = case shown="False" w173 {
          tunnel: [u32 4664063 u32 11796992] -> w172
          frame False {
          }
          frame True {
          }
        }
        n161 = case shown="False" w171 {
          tunnel: [u32 4664063 u32 11796992] -> w170
          frame False {
          }
          frame True {
          }
        }
        n162 = local read "Config Cluster"() -> (w161:T7)
        n163 = Unbundle By Name(w161) -> ("Scale Position High Offset"=w99:dbl, "Intake Position Offset"=w100:dbl)
        n164 = property on="FL Spin" class="Knob (strict)"("FG Color"=w175) -> ()  [unwired: 2 in, 2 out]
        n165 = property on="FR Spin" class="Knob (strict)"("FG Color"=w172) -> ()  [unwired: 2 in, 2 out]
        n166 = property on="BL Spin" class="Knob (strict)"("FG Color"=w170) -> ()  [unwired: 2 in, 2 out]
        n167 = property on="BR Spin" class="Knob (strict)"("FG Color"=w169) -> ()  [unwired: 2 in, 2 out]
        n168 = call "Lift Fill Select.vi"("Trigger Buffer"=6000.0, "Lift Ref Point"=w111, "Lift Position"=w112, "Config Cluster"=w161) -> ("Fill Color"=w165:dbl)  [unwired: 7 in]
        n169 = Cluster To Array(cluster=w161) -> (array=w198:dbl[])
        n170 = And(x="Read Sheet 2", y="Arm Read Config") -> (x .and. y?=w194:bool)
        n171 = And(x="Arm Write Config", y="Write to Sheet 2") -> (x .and. y?=w193:bool)
        n172 = case shown="8" w165 {
          tunnel: [u32 0 u32 13107968 u32 14446080 u32 15716352 u32 9895680 u32 14847 u32 11534591 u32 16722652 u32 16746675] -> w167
          frame 0, Default {
          }
          frame 1 {
          }
          frame 2 {
          }
          frame 3 {
          }
          frame 4 {
          }
          frame 5 {
          }
          frame 6 {
          }
          frame 7 {
          }
          frame 8 {
          }
        }
        n173 = Subtract(x=w99, y=w100) -> (x-y=w101:dbl)
        n174 = Add(x=w100, y=w111) -> (x+y=w159:dbl)
        n175 = case shown="True" w194 {
          tunnel: "Config Cluster File Path" -> [_ w346]
          tunnel: [FALSE TRUE] -> w196
          frame False {
          }
          frame True {
            n176 = call-poly <vilib>:"Read Delimited Spreadsheet.vi"("file path (dialog if empty)"=w346, "format (%.3f)"="%g", "delimiter (\\t)"="," ("delimiter (\\t)")) -> ("first row"=w342:dbl[])  [unwired: 7 in, 5 out]
            n177 = Array To Cluster(array=w342) -> (cluster=w340:T13)
            n178 = local write "Arm Read Config"(FALSE ("Update\nDB Table")) -> ()
            n179 = local write "Config Cluster"(w340) -> ()
          }
        }
        n180 = case shown="True" w193 {
          tunnel: "Config Cluster File Path" -> [_ w351]
          tunnel: [FALSE ("Saved to Sheet") TRUE ("Saved to Sheet")] -> w195
          tunnel: w198 -> [_ w349]
          frame False {
          }
          frame True {
            n181 = call-poly <vilib>:"Write Delimited Spreadsheet.vi"("file path (dialog if empty)"=w351, "format (%.3f)"="%g", "1D data"=w349, "delimiter (\\t)"="," ("delimiter (\\t)")) -> ()  [unwired: 10 in, 2 out]
          }
        }
        n182 = Subtract(x=w112, y=w159) -> (x-y=→"Lift Position":dbl)
        n183 = property on="Lift Position" class="Slide (strict)"("Fill Color"=w167, "Scale.Maximum"=w101) -> ()  [unwired: 2 in, 2 out]
        n184 = call-poly <vilib>:"NT Write Value.vi"("Numeric Array"=w198, "Name"="Config") -> ()  [unwired: 9 in, 1 out]
        n185 = Build Array("Save Zeros to File", "Read Zeros from File", "Zero Drive", "Zero FL", "Zero FR", "Zero BL", "Zero BR") -> (w183:bool[])
        n186 = case shown="True" w195 {
          tunnel: [cluster{u32, u32}[] [{1985280, 0}, {16750592, 0}] ("Colors [4]") cluster{u32, u32}[] [{1985280, 0}, {6618880, 0}] ("Colors [4]")] -> w201
          frame True {
          }
          frame False {
          }
        }
        n187 = case shown="True" "Enable Zero Ctrls" {
          tunnel: [bool[] [] w338] -> w184
          tunnel: w183 -> [_ w338]
          frame False {
          }
          frame True {
          }
        }
        n188 = Or(x=w195, y=w196) -> (x .or. y?=→"Feedback 2":bool)
        n189 = call-poly <vilib>:"NT Read Value.vi"("Name"="Intake Short" ("refnum name")) -> ("Boolean"=→"Intake Short":bool)  [unwired: 9 in, 1 out]
        n190 = call-poly <vilib>:"NT Read Value.vi"("Name"="Drive Orientation") -> ("Boolean"=→"Drive Orientation":bool)  [unwired: 9 in, 1 out]
        n191 = call-poly <vilib>:"NT Read Value.vi"("Name"="Intake Long" ("refnum name")) -> ("Boolean"=→"Intake Long":bool)  [unwired: 9 in, 1 out]
        n192 = call-poly <vilib>:"NT Read Value.vi"("Default Value"=TRUE, "Name"="Ramp Tail" ("refnum name")) -> ("Boolean"=→"Ramp Tail Status":bool)  [unwired: 8 in, 1 out]
        n193 = Select(t=T14."Enabled" ("Disabled"), s="Enable Zero Ctrls", f=T14."Disabled and Grayed Out" ("Disabled")) -> (s? t:f=w143:T14)
        n194 = call-poly <vilib>:"NT Write Value.vi"("Boolean Array"=w184, "Name"="Swerve Bool Config") -> ()  [unwired: 9 in, 1 out]
        n195 = property on="Feedback 2" class="Bool (strict)"("Colors [4]"=w201) -> ()  [unwired: 2 in, 2 out]
        n196 = property on="Read Zeros from File" class="Bool (strict)"("DisabledEnum"=w143) -> ()  [unwired: 2 in, 2 out]
        n197 = property on="Save Zeros to File" class="Bool (strict)"("DisabledEnum"=w143) -> ()  [unwired: 2 in, 2 out]
        n198 = property on="Zero Drive" class="Bool (strict)"("DisabledEnum"=w143) -> ()  [unwired: 2 in, 2 out]
        n199 = call-poly <vilib>:"NT Read Value.vi"("Name"="Auto Frame Status") -> ("Numeric"=→"Auto Frame":dbl)  [unwired: 9 in, 1 out]
        n200 = call-poly <vilib>:"NT Read Value.vi"("Name"="Swerve Zero Feedback") -> ("Boolean"=→"Control Feedback":bool)  [unwired: 9 in, 1 out]
        n201 = call-poly <vilib>:"NT Read Value.vi"("Name"="Zero Feedback") -> ("Boolean"=→"Zero Feedback":bool)  [unwired: 9 in, 1 out]
        n202 = property on="Zero FL" class="Bool (strict)"("DisabledEnum"=w143) -> ()  [unwired: 2 in, 2 out]
        n203 = case shown="False" "Flush Network Table" {
          tunnel: [FALSE TRUE] -> w116
          frame False {
          }
          frame True {
            n204 = call <vilib>:"NT Flush Data Updates.vi"() -> ()  [unwired: 11 in, 1 out]
          }
        }
        "Flush feedback" <- w116
        n205 = property on="Zero FR" class="Bool (strict)"("DisabledEnum"=w143) -> ()  [unwired: 2 in, 2 out]
        n206 = property on="Zero BL" class="Bool (strict)"("DisabledEnum"=w143) -> ()  [unwired: 2 in, 2 out]
        n207 = property on="Zero BR" class="Bool (strict)"("DisabledEnum"=w143) -> ()  [unwired: 2 in, 2 out]
        n208 = call-poly <vilib>:"NT Write Value.vi"("Boolean"="Reset Lift to Start Config", "Name"="Zero Lift") -> ()  [unwired: 9 in, 1 out]
        n209 = call-poly <vilib>:"NT Write Value.vi"("Boolean"="Zero Gyro", "Name"="Zero Gyro") -> ()  [unwired: 9 in, 1 out]
      }
    }
  }
  n210 = Bundle("Camera Image"=w55, "Dashboard Tab"=w54, "Background"=w50, "Rec Mode"=w43, "Test Slider"=w42, "On/Off"=w41, "Test Ring"=w40, "Rev/Fwd"=w39, "Test Name"=w45, "Motor"=w44, "Progress"=w38, "CheckList"=w48, "Tree"=w47, "Test Tree"=w46, "Command Params"=w32, "Command Selection"=w29, "Execute Command"=w31, "Cmd Status"=w25, "Camera Settings"=w21, "Camera Name"=w20, "Camera Info"=w19, "Camera Settings Right"=w9, "Camera Name Right"=w8, "Camera Image Right"=w7) -> (w49:T23)  [unwired: 1 in]
  n211 = call "Handle Camera Configuration.vi"("CameraNameRef"=w22, "Display Name"=w2, "ClusterRef"=w23) -> ()  [unwired: 9 in]
  n212 = while {
    tunnel: w75 -> [w407]
    tunnel: w74 -> [_]
    tunnel: [w408] -> _
    tunnel: w4 -> [w398]
    tunnel: w2 -> [w395]
    i -> [w408]
    stop <- FALSE stop-if-true
    # "Optionally read the DB image,\nlog, or retrieve images from a\nlogged match"
    n213 = local read "NT Connection"() -> (w399:bool)
    n214 = local read "Rec Mode"() -> (w403:enum32{"Stop", "Record", "Playback"})
    n215 = Bundle("Camera Name"="Camera Name", w395, "Saved DB Images Info"=w398) -> (w397:T24)  [unwired: 1 in]
    n216 = call <vilib>:"WPI_CameraRead MJPG for Dashboard.vi"("Camera Settings"="Camera Settings", "Rec Mode"=w403, "NT Connection"=w399, "Capture Info"=w397, "Refnum in"=w407) -> ("Active"=w405:bool, "Refnum out"=w406:T5, "FPS"=w404:dbl, "Bandwidth (Mbps)"=w402:dbl)  [unwired: 3 in]
    n217 = case shown="True" w405 {
      tunnel: w406 -> [w410 w421]
      tunnel: w402 -> [_ w418]
      tunnel: w404 -> [_ w419]
      tunnel: [w410 w415] -> w400
      frame False {
        w412 = u32 1985280 ("Color Box")
        # "Sleep for 500ms"
        n218 = Bundle("Color Box"=w412, "Color Box"=w412) -> (w413:cluster{"Color Box":u32, "Color Box":u32})  [unwired: 1 out]
        n219 = Build Array(w413) -> (w411:cluster{"Color Box":u32, "Color Box":u32}[])
        n220 = property on="Mbps LED" class="Bool (strict)"("Colors [4]"=w411) -> ()  [unwired: 2 in, 2 out]
        n221 = Wait Until Next ms Multiple(millisecond multiple=u32 500) -> ()  [unwired: 1 out]
      }
      frame True {
        # "Here is where you would annotate,\npossibly process, and display the image"
        # "Update Mbps LED"
        n222 = case shown="Default" w418 {
          tunnel: [u32 6618880 ("Color Box") u32 16776722 ("Color Box") u32 16716800 ("Color Box")] -> w422
          frame Default {
          }
          frame 4, 5 {
          }
          frame 6.. {
          }
        }
        n223 = call "IMAQ Clear Overlay"("Image"=w421) -> ("error out"=w424:errorcluster, "Image Out"=w415:T5)  [unwired: 2 in, 7 out]
        n224 = Bundle(FALSE, "Bandwidth (Mbps)"=w418, "FPS"=w419) -> (→"Camera Info":cluster{bool, "Bandwidth (Mbps)":dbl, "FPS":dbl})  [unwired: 1 in]
        n225 = Bundle("Color Box"=w422, "Color Box"=w422) -> (w423:cluster{"Color Box":u32, "Color Box":u32})  [unwired: 1 out]
        n226 = Unbundle By Name(w424) -> ("status"=w425:bool)
        n227 = Build Array(w423) -> (w420:cluster{"Color Box":u32, "Color Box":u32}[])
        n228 = property on="Image Message" class="Str"("Visible"=w425) -> ()  [unwired: 2 in, 2 out]
        n229 = property on="Mbps LED" class="Bool (strict)"("Colors [4]"=w420) -> ()  [unwired: 2 in, 2 out]
      }
    }
    "Camera Image" <- w400
  }
  n230 = call "Handle Camera Configuration.vi"("CameraNameRef"=w10, "Display Name"=w3, "ClusterRef"=w11) -> ()  [unwired: 9 in]
  n231 = while {
    tunnel: w13 -> [w443]
    tunnel: w12 -> [_]
    tunnel: [w438] -> _
    tunnel: w4 -> [w432]
    tunnel: w3 -> [w429]
    i -> [w438]
    stop <- FALSE stop-if-true
    n232 = local read "NT Connection"() -> (w433:bool)
    n233 = local read "Rec Mode"() -> (w442:enum32{"Stop", "Record", "Playback"})
    n234 = Bundle("Camera Name Right"="Camera Name Right", w429, "Saved DB Images Info"=w432) -> (w431:T25)  [unwired: 1 in]
    n235 = call <vilib>:"WPI_CameraRead MJPG for Dashboard.vi"("Camera Settings"="Camera Settings Right", "Rec Mode"=w442, "NT Connection"=w433, "Capture Info"=w431, "Refnum in"=w443) -> ("Active"=w437:bool, "Refnum out"=w440:T5, "FPS"=w435:dbl, "Bandwidth (Mbps)"=w436:dbl)  [unwired: 3 in]
    n236 = case shown="False" w437 {
      tunnel: w440 -> [w444 w446]
      tunnel: w436 -> [_ _]
      tunnel: w435 -> [_ _]
      tunnel: [w444 w446] -> w434
      frame False {
        n237 = Wait Until Next ms Multiple(millisecond multiple=u32 500) -> ()  [unwired: 1 out]
      }
      frame True {
      }
    }
    "Camera Image Right" <- w434
  }
  n238 = register-events(refnum<vi> refnum, w26) -> (reference out=w64:refnum<event-registration>, error out=w63:errorcluster)  [unwired: 2 in]
  n239 = call "Initialize Camera and CheckList.vi"("ListBox in"=w48) -> ()  [unwired: 11 in]
  n240 = call "Adjust Dashboard Window.vi"("Sizing Refnums"=w49, "Size Constraints"=w51, "VI"=w59, "WIn Mode"=w35) -> ()  [unwired: 8 in]
  n241 = while {
    tunnel: w56 -> [w458]
    tunnel: w36 -> [w456]
    tunnel: [w454] -> _
    tunnel: u32 1000 ("milliseconds to wait") -> [w453]
    tunnel: w26 -> [w447]
    i -> [w454]
    stop <- FALSE stop-if-true
    n242 = local read "Rec Mode"() -> (w449:enum32{"Stop", "Record", "Playback"})
    n243 = Wait on Notification(notifier=w456, timeout in ms (-1)=w453) -> (notification=w455:string, timed out?=w451:bool)  [unwired: 2 in, 2 out]
    n244 = Equal?(x=w449, y=u16 2 ("Rec Mode")) -> (x = y?=w450:bool)
    n245 = Compound Arithmetic op=OR(invert w451, w450) -> (w452:bool)
    n246 = case shown="True" w452 {
      tunnel: w458 -> [_ w461]
      tunnel: w455 -> [_ w460]
      tunnel: w447 -> [_ w459]
      frame False {
      }
      frame True {
        n247 = call <vilib>:"Bind Controls to SmartDashboard.vi"("RPC ref"=w459, "Bound Control Refs"=w461, "Server IP Address"=w460) -> ()  [unwired: 9 in]
      }
    }
  }
  n248 = vi-ref "Playback Controls.vi"() -> (w65:refnum<vi>)
  n249 = property class="VI"() -> ("Panel"=w67:refnum<vi>)  [unwired: 2 in, 2 out]
  n250 = property class="Pnl"(reference=w67) -> ("Panes[]"=w68:refnum<vi>[])  [unwired: 1 in, 2 out]
  n251 = Index Array(array=w68) -> (element=w66:refnum<vi>)  [unwired: 1 in]
  n252 = control-ref of="Test Tree"() -> (w69:refnum<vi>)
  n253 = while {
    tunnel: [w471] -> _
    tunnel: w69 -> [w470]
    tunnel: w65 -> [w469]
    tunnel: w64 -> [w468]
    tunnel: w63 -> [_]
    tunnel: w59 -> [w467]
    tunnel: w26 -> [w466]
    tunnel: w24 -> [w465]
    shift-right: [w464] -> _
    shift-left: _ -> [w463]
    tunnel: w18 -> [w462]
    i -> [w471]
    stop <- FALSE stop-if-true
    n254 = event shown="[0] Timeout" {
      selector: w468 -> [_ _ _ _ _ _ _ _ _ _ _ _ _ _ _ _ _ _ _ _ _]
      dyn-events: [_ _ _ _ _ _ _ _ _ _ _ _ _ _ _ _ w731 _ _ _ _] -> _
      timeout: u32 60 ("milliseconds to wait") -> [_ _ _ _ _ _ _ _ _ _ _ _ _ _ _ _ _ _ _ _ _]
      tunnel: w470 -> [w483 _ _ _ _ _ _ _ _ _ _ _ _ _ _ _ _ _ _ _ _]
      tunnel: "Test Tree" -> [_ _ _ _ _ _ _ _ _ _ _ w698 w706 w708 w712 w720 _ _ _ _ _]
      tunnel: w469 -> [_ _ _ _ _ _ _ _ _ _ _ _ _ _ _ _ w733 _ w751 _ _]
      tunnel: w467 -> [_ _ _ _ _ _ _ _ _ _ _ _ _ _ _ _ w729 _ _ _ _]
      tunnel: w466 -> [_ _ _ _ _ _ _ _ _ _ _ _ _ _ _ _ w727 _ _ _ _]
      tunnel: w465 -> [w478 _ _ _ _ _ w649 _ _ _ _ _ _ _ _ _ _ _ _ _ _]
      tunnel: [w477 w526 w628 w633 w642 w646 w647 w656 w666 w673 w685 w697 w704 w707 w711 w719 w726 w746 w748 w752 w765] -> w464
      tunnel: w463 -> [w477 w526 w628 w633 w642 w646 w647 _ _ w673 w685 w697 w704 w707 w711 w719 w726 w746 w748 w752 w765]
      tunnel: w462 -> [w475 _ _ _ _ _ _ _ _ _ _ _ _ _ _ _ _ _ _ _ _]
      event Timeout {
        n255 = event-data() -> ()  [unwired: 1 in, 1 out]
        n256 = local read "Mode"() -> (w480:T4)
        n257 = case shown="\"Commands\"" "Dashboard Tab" {
          tunnel: w483 -> [_ _ w499 _ _]
          tunnel: "TestMode/Automatic/" ("Name Pattern") -> [_ _ w498 _ _]
          tunnel: T26 [{"Operation"=enum."Clear", "Color Box"=14013909}, {"Operation"=enum."Clear", "Color Box"=14013909}, {"Operation"=enum."Clear", "Color Box"=14013909}, {"Operation"=enum."Clear", "Color Box"=14013909}, {"Operation"=enum."Update", "Color Box"=14013909}, {"Operation"=enum."Update", "Color Box"=16777215}, {"Operation"=enum."Clear", "Color Box"=14013909}, {"Operation"=enum."Clear", "Color Box"=14013909}, {"Operation"=enum."Clear", "Color Box"=14013909}] -> [_ _ w491 _ w519]
          tunnel: w480 -> [_ _ w490 _ w518]
          tunnel: u32[] [15790320, 15790320, 15790320, 15790320, 16777215, 16777215, 15790320, 15790320, 15790320] -> [_ _ _ _ w524]
          tunnel: w478 -> [_ _ _ _ w512]
          tunnel: w475 -> [_ w485 _ _ _]
          frame "Auto", Default {
          }
          frame "Drive" {
            n258 = call <vilib>:"WPI_DashboardUpdateNames.vi"("Controls on Tab"=w485) -> ()  [unwired: 11 in]
          }
          frame "Test" {
            w497 = -2 ("Active Item:Row Number")
            n259 = Index Array(array=w491, index=w490) -> (element=w492:T29)
            n260 = Unbundle(w492) -> ("Operation"=w493:enum16{"Update", "Clear"}, "Color Box"=w494:u32)
            n261 = call <vilib>:"NT Read String.vi"("Name"="TestMode/TestName") -> ("String"=w488:string)  [unwired: 9 in, 1 out]
            n262 = call <vilib>:"NT Read and Format Entries as Tree.vi"("Operation"=w493, "Name Pattern"=w498, "Tree Refnum"=w499) -> ()  [unwired: 7 in, 2 out]
            n263 = case shown="\"\"" w488 {
              tunnel: "TestMode/TestProgress" ("Name") -> [w501 _]
              tunnel: "TestMode/TestProgressText" ("Name") -> [w500 _]
              frame Default {
                n264 = call <vilib>:"NT Read Number.vi"("Name"=w501) -> ("Numeric"=w502:dbl)  [unwired: 9 in, 1 out]
                n265 = call <vilib>:"NT Read String.vi"("Name"=w500) -> ("String"=w503:string)  [unwired: 9 in, 1 out]
                n266 = Bundle("Numeric"=w502, "String"=w503) -> (→"Progress":cluster{"Numeric":dbl, "String":string})  [unwired: 1 in]
              }
              frame "" {
                n267 = property on="Progress" class="Clust (strict)"("Visible"=FALSE) -> ()  [unwired: 2 in, 2 out]
                n268 = local write "Test Name"(u16 0) -> ()
              }
            }
            n269 = property on="Test Tree" class="Tree (strict)"("Active Item Row Number"=w497, "ActiveColNum"=w497, "CellBG"=w494, "Active Item Row Number"=-1 ("Active Item:Row Number"), "CellBG"=u32 5789784 ("Color Box")) -> ()  [unwired: 2 in, 2 out]
          }
          frame "Variables" {
            w509 = string[] ["CameraPublisher", "Usage", "DB"]  # Items to initially close
            n270 = First Call?() -> (First Call?: T/F=w510:bool)
            n271 = control-ref of="Tree"() -> (w511:refnum<vi>)
            n272 = Select(t=w509, s=w510, f=string[] []) -> (s? t:f=w507:string[])
            n273 = call <vilib>:"NT Read and Format Entries as Tree.vi"("Tags to  Close"=w507, "Tree Refnum"=w511) -> ()  [unwired: 8 in, 2 out]
          }
          frame "Commands" {
            w520 = u32 5789784 ("Color Box")
            w521 = T30 {"Row"=-1, "Column"=-2} ("Active Cell:Active Cell")
            w523 = T30 {"Row"=-2, "Column"=-2} ("Active Cell:Active Cell")
            n274 = Index Array(array=w524, index=w518) -> (element=w522:u32)
            n275 = Index Array(array=w519, index=w518) -> (element=w517:T29)
            n276 = Unbundle(w517) -> ("Operation"=w516:enum16{"Update", "Clear"})  [unwired: 1 out]
            n277 = local read "Command Selection"() -> (w515:i32)
            n278 = property on="Command Selection" class="MCListbox (strict)"("ActiveCell"=w523, "CellBG"=w522, "ActiveCell"=w521, "CellBG"=w520) -> ()  [unwired: 2 in, 2 out]
            n279 = call <vilib>:"WPI_DashboardUpdate RPC Info.vi"("Operation"=w516) -> ("update"=w514:bool, "commands"=w513:string[][])  [unwired: 9 in]
            n280 = property on="Command Selection" class="MCListbox (strict)"("ItemNames"=w513) -> ()  [unwired: 2 in, 2 out]
            n281 = property on="Command Params" class="Tbl (strict)"("Active Cell"=w523, "Cell BG Color"=w522, "Active Cell"=w521, "Cell BG Color"=w520) -> ()  [unwired: 2 in, 2 out]
            n282 = call <vilib>:"WPI_DashboardUpdate Command Params.vi"("Update"=w514, "NewVal"=w515, "Commands"=w513, "Param Tbl"=w512) -> ()  [unwired: 7 in, 1 out]
          }
        }
        n283 = call <vilib>:"Connextion Info.vi"() -> ("Connected"=→"NT Connection":bool)  [unwired: 10 in, 1 out]
      }
      event "Test Tree": Value Change {
        # "Show appropriate\ncontrols"
        n284 = event-data() -> ("CtlRef"=w529:refnum<vi>, "NewVal"=w527:string)  [unwired: 1 in]
        n285 = call <vilib>:"WPI_UtilitiesGetTreeIOName.vi"("NewVal"=w527, "TreeControl in"=w529) -> ("I/O Name"=w530:string)  [unwired: 9 in]
        n286 = case shown="\"Camera\"" w530 {
          selector: w530 -> [_ w537 _ w559 w568 _]
          tunnel: w527 -> [_ _ w556 w558 _ w575]
          tunnel: cluster{string[]}[] [{["640x480", "320x240", "160x120"]}, {["Auto", "Fixed indoor", "Fixed outdoor 1", "Fixed outdoor 2", "Fixed fluorescent 1", "Fixed fluorescent 2", "Hold current"]}, {["Auto", "Flicker-free 50 Hz", "Flicker-free 60 Hz", "Hold current"]}, {["None", "Prioritize frame rate", "Prioritize image quality"]}, {["Monochrome", "Color"]}] -> [_ _ _ _ _ w574]
          frame Default {
            w532 = FALSE ("Visible")
            w531 = FALSE ("Visible")
            n287 = property on="Motor" class="Clust (strict)"("Visible"=w531) -> ()  [unwired: 2 in, 2 out]
            n288 = property on="Test Ring" class="Ring (strict)"("Visible"=w531) -> ()  [unwired: 2 in, 2 out]
            n289 = property on="Rev/Fwd" class="Clust (strict)"("Visible"=w532) -> ()  [unwired: 2 in, 2 out]
            n290 = property on="On/Off" class="Bool (strict)"("Visible"=w532) -> ()  [unwired: 2 in, 2 out]
            n291 = property on="Test Slider" class="Slide (strict)"("Visible"=w532) -> ()  [unwired: 2 in, 2 out]
          }
          frame "Analog Out", "Motor", "PWM" {
            w538 = FALSE ("Visible")
            n292 = case shown="\"Analog Out\"" w537 {
              tunnel: [1.0 ("Value") -1.0 ("Value") 0.0 ("Value")] -> w536
              tunnel: [255.0 ("Value") 1.0 ("Value") 5.0 ("Value")] -> w535
              tunnel: [128.0 ("Value") 0.0 ("Value") 0.0 ("Value")] -> w534
              tunnel: [64.0 ("Value") 0.5 ("Value") 1.0 ("Value")] -> w533
              frame "PWM" {
              }
              frame "Motor", Default {
              }
              frame "Analog Out" {
              }
            }
            n293 = property on="Motor" class="Clust (strict)"("Visible"=TRUE) -> ()  [unwired: 2 in, 2 out]
            n294 = property on="Value" class="Slide (strict)"("Value"=w534, "Scale.Minimum"=w536, "Scale.Maximum"=w535, "Scale.Increment"=w533) -> ()  [unwired: 2 in, 2 out]
            n295 = property on="On/Off" class="Bool (strict)"("Visible"=w538) -> ()  [unwired: 2 in, 2 out]
            n296 = property on="Test Slider" class="Slide (strict)"("Visible"=w538) -> ()  [unwired: 2 in, 2 out]
            n297 = property on="Test Ring" class="Ring (strict)"("Visible"=w538) -> ()  [unwired: 2 in, 2 out]
            n298 = property on="Rev/Fwd" class="Clust (strict)"("Visible"=w538) -> ()  [unwired: 2 in, 2 out]
          }
          frame "Servo" {
            w554 = FALSE ("Visible")
            n299 = call <vilib>:"NT Read Number.vi"("Name"=w556) -> ("Numeric"=w555:dbl)  [unwired: 9 in, 1 out]
            n300 = property on="Test Slider" class="Slide (strict)"("Visible"=TRUE, "Scale.Maximum"=170.0 ("Scale.Range:Maximum")) -> ()  [unwired: 2 in, 2 out]
            n301 = local write "Test Slider"(w555) -> ()
            n302 = property on="Motor" class="Clust (strict)"("Visible"=w554) -> ()  [unwired: 2 in, 2 out]
            n303 = property on="Rev/Fwd" class="Clust (strict)"("Visible"=w554) -> ()  [unwired: 2 in, 2 out]
            n304 = property on="On/Off" class="Bool (strict)"("Visible"=w554) -> ()  [unwired: 2 in, 2 out]
            n305 = property on="Test Ring" class="Ring (strict)"("Visible"=w554) -> ()  [unwired: 2 in, 2 out]
          }
          frame "Relay", "Solenoid" {
            w557 = FALSE ("Visible")
            n306 = property on="Motor" class="Clust (strict)"("Visible"=w557) -> ()  [unwired: 2 in, 2 out]
            n307 = property on="Test Slider" class="Slide (strict)"("Visible"=w557) -> ()  [unwired: 2 in, 2 out]
            n308 = Search and Replace String(input string=w558, search string="/Value  **", replace string="/Direction") -> (result string=w564:string)  [unwired: 5 in, 3 out]
            n309 = property on="Test Ring" class="Ring (strict)"("Visible"=w557) -> ()  [unwired: 2 in, 2 out]
            n310 = call <vilib>:"NT Read String.vi"("Name"=w564) -> ("String"=w562:string)  [unwired: 9 in, 1 out]
            n311 = Equal?(x="Both directions", y=w562) -> (x = y?=w560:bool)
            n312 = Not(x=w560) -> (.not. x?=w561:bool)
            n313 = property on="Rev/Fwd" class="Clust (strict)"("Visible"=w560) -> ()  [unwired: 2 in, 2 out]
            n314 = property on="On/Off" class="Bool (strict)"("Visible"=w561, "Caption.Text"=w559) -> ()  [unwired: 2 in, 2 out]
          }
          frame "Compressor", "Digital Out" {
            w567 = FALSE ("Visible")
            # "Get direction and finish"
            n315 = property on="Motor" class="Clust (strict)"("Visible"=w567) -> ()  [unwired: 2 in, 2 out]
            n316 = property on="Test Slider" class="Slide (strict)"("Visible"=w567) -> ()  [unwired: 2 in, 2 out]
            n317 = property on="Test Ring" class="Ring (strict)"("Visible"=w567) -> ()  [unwired: 2 in, 2 out]
            n318 = property on="On/Off" class="Bool (strict)"("Visible"=TRUE, "Caption.Text"=w568) -> ()  [unwired: 2 in, 2 out]
            n319 = property on="Rev/Fwd" class="Clust (strict)"("Visible"=FALSE) -> ()  [unwired: 2 in, 2 out]
          }
          frame "Camera" {
            n320 = call <vilib>:"Get Last Path Segment.vi"("String in"=w575) -> ("String out"=w576:string)  [unwired: 10 in]
            n321 = property on="On/Off" class="Bool (strict)"("Visible"=FALSE) -> ()  [unwired: 2 in, 2 out]
            n322 = property on="Motor" class="Clust (strict)"("Visible"=FALSE) -> ()  [unwired: 2 in, 2 out]
            n323 = property on="Rev/Fwd" class="Clust (strict)"("Visible"=FALSE) -> ()  [unwired: 2 in, 2 out]
            n324 = case shown="\"White Balance  **\"" w576 {
              tunnel: w575 -> [w582 w591 w600 w609 w618 _ w624]
              tunnel: w574 -> [w580 w588 w597 w606 w615 _ _]
              frame "Size  **" {
                n325 = Index Array(array=w580) -> (element=w579:cluster{string[]})  [unwired: 1 in]
                n326 = call <vilib>:"NT Read String.vi"("Name"=w582) -> ("String"=w581:string)  [unwired: 9 in, 1 out]
                n327 = Unbundle(w579) -> (w577:string[])
                n328 = Match First String(2:w577, 3:w581) -> (0:w578:i32)  [unwired: 1 out]
                n329 = property on="Test Ring" class="Ring (strict)"("Value"=w578, "Strings []"=w577) -> ()  [unwired: 2 in, 2 out]
                n330 = property on="Test Ring" class="Ring (strict)"("Visible"=TRUE) -> ()  [unwired: 2 in, 2 out]
                n331 = property on="Test Slider" class="Slide (strict)"("Visible"=FALSE) -> ()  [unwired: 2 in, 2 out]
              }
              frame "White Balance  **" {
                n332 = Index Array(array=w588, index=1) -> (element=w589:cluster{string[]})
                n333 = call <vilib>:"NT Read String.vi"("Name"=w591) -> ("String"=w590:string)  [unwired: 9 in, 1 out]
                n334 = Unbundle(w589) -> (w586:string[])
                n335 = Match First String(2:w586, 3:w590) -> (0:w585:i32)  [unwired: 1 out]
                n336 = property on="Test Ring" class="Ring (strict)"("Value"=w585, "Strings []"=w586) -> ()  [unwired: 2 in, 2 out]
                n337 = property on="Test Ring" class="Ring (strict)"("Visible"=TRUE) -> ()  [unwired: 2 in, 2 out]
                n338 = property on="Test Slider" class="Slide (strict)"("Visible"=FALSE) -> ()  [unwired: 2 in, 2 out]
              }
              frame "Exposure  **" {
                n339 = Index Array(array=w597, index=2) -> (element=w598:cluster{string[]})
                n340 = call <vilib>:"NT Read String.vi"("Name"=w600) -> ("String"=w599:string)  [unwired: 9 in, 1 out]
                n341 = Unbundle(w598) -> (w594:string[])
                n342 = Match First String(2:w594, 3:w599) -> (0:w595:i32)  [unwired: 1 out]
                n343 = property on="Test Ring" class="Ring (strict)"("Value"=w595, "Strings []"=w594) -> ()  [unwired: 2 in, 2 out]
                n344 = property on="Test Ring" class="Ring (strict)"("Visible"=TRUE) -> ()  [unwired: 2 in, 2 out]
                n345 = property on="Test Slider" class="Slide (strict)"("Visible"=FALSE) -> ()  [unwired: 2 in, 2 out]
              }
              frame "Exposure Priority  **" {
                n346 = Index Array(array=w606, index=3) -> (element=w607:cluster{string[]})
                n347 = call <vilib>:"NT Read String.vi"("Name"=w609) -> ("String"=w608:string)  [unwired: 9 in, 1 out]
                n348 = Unbundle(w607) -> (w603:string[])
                n349 = Match First String(2:w603, 3:w608) -> (0:w604:i32)  [unwired: 1 out]
                n350 = property on="Test Ring" class="Ring (strict)"("Value"=w604, "Strings []"=w603) -> ()  [unwired: 2 in, 2 out]
                n351 = property on="Test Ring" class="Ring (strict)"("Visible"=TRUE) -> ()  [unwired: 2 in, 2 out]
                n352 = property on="Test Slider" class="Slide (strict)"("Visible"=FALSE) -> ()  [unwired: 2 in, 2 out]
              }
              frame "Color Enable  **" {
                n353 = Index Array(array=w615, index=4) -> (element=w616:cluster{string[]})
                n354 = call <vilib>:"NT Read String.vi"("Name"=w618) -> ("String"=w617:string)  [unwired: 9 in, 1 out]
                n355 = Unbundle(w616) -> (w612:string[])
                n356 = Match First String(2:w612, 3:w617) -> (0:w613:i32)  [unwired: 1 out]
                n357 = property on="Test Ring" class="Ring (strict)"("Value"=w613, "Strings []"=w612) -> ()  [unwired: 2 in, 2 out]
                n358 = property on="Test Ring" class="Ring (strict)"("Visible"=TRUE) -> ()  [unwired: 2 in, 2 out]
                n359 = property on="Test Slider" class="Slide (strict)"("Visible"=FALSE) -> ()  [unwired: 2 in, 2 out]
              }
              frame Default {
                n360 = property on="Test Ring" class="Ring (strict)"("Visible"=FALSE) -> ()  [unwired: 2 in, 2 out]
                n361 = property on="Test Slider" class="Slide (strict)"("Visible"=FALSE) -> ()  [unwired: 2 in, 2 out]
              }
              frame "Brightness  **", "Color Level  **", "Compression  **", "FPS  **", "Sharpness  **" {
                n362 = call <vilib>:"NT Read Number.vi"("Name"=w624) -> ("Numeric"=w623:dbl)  [unwired: 9 in, 1 out]
                n363 = local write "Test Slider"(w623) -> ()
                n364 = property on="Test Slider" class="Slide (strict)"("Visible"=TRUE, "Scale.Maximum"=100.0 ("Scale.Range:Maximum")) -> ()  [unwired: 2 in, 2 out]
                n365 = property on="Test Ring" class="Ring (strict)"("Visible"=FALSE) -> ()  [unwired: 2 in, 2 out]
              }
            }
          }
        }
        n366 = property on="Progress" class="Clust (strict)"("Visible"=FALSE) -> ()  [unwired: 2 in, 2 out]
      }
      event "Test Name": Mouse Enter {
        # "Populate the ring with the list of tests"
        n367 = event-data() -> ()  [unwired: 1 in, 1 out]
        n368 = call <vilib>:"NT Read String Array.vi"("Name"="TestMode/TestList") -> ("String Array"=w632:string[])  [unwired: 9 in, 1 out]
        n369 = Build Array (concatenate)("Select the test to run...", w632) -> (w631:string[])
        n370 = property on="Test Name" class="Ring (strict)"("Strings []"=w631) -> ()  [unwired: 2 in, 2 out]
      }
      event "Test Name": Value Change {
        w634 = FALSE ("Visible")
        # "Tell the robot the test name to run"
        n371 = event-data() -> ("NewVal"=w638:u16)  [unwired: 1 in]
        n372 = property on="Test Name" class="Ring (strict)"() -> ("Strings []"=w639:string[])  [unwired: 2 in, 2 out]
        n373 = local write "Progress"(T8 {"Test Progress"=0, "Test Progress Text"=""} ("Progress")) -> ()
        n374 = Index Array(array=w639, index=w638) -> (element=w637:string)
        n375 = call <vilib>:"NT Write String.vi"("String"=w637, "Name"="TestMode/TestName") -> ()  [unwired: 9 in, 1 out]
        n376 = property on="Progress" class="Clust (strict)"("Visible"=TRUE) -> ()  [unwired: 2 in, 2 out]
        n377 = property on="Motor" class="Clust (strict)"("Visible"=w634) -> ()  [unwired: 2 in, 2 out]
        n378 = property on="Test Slider" class="Slide (strict)"("Visible"=w634) -> ()  [unwired: 2 in, 2 out]
        n379 = property on="On/Off" class="Bool (strict)"("Visible"=w634) -> ()  [unwired: 2 in, 2 out]
        n380 = property on="Rev/Fwd" class="Clust (strict)"("Visible"=w634) -> ()  [unwired: 2 in, 2 out]
        n381 = property on="Test Ring" class="Ring (strict)"("Visible"=w634) -> ()  [unwired: 2 in, 2 out]
      }
      event "Select Auto": Mouse Enter {
        # "Populate the combo box with the list of autonomous options"
        n382 = event-data() -> ()  [unwired: 1 in, 1 out]
        n383 = call <vilib>:"NT Read String Array.vi"("Name"="Auto List") -> ("String Array"=w641:string[])  [unwired: 9 in, 1 out]
        n384 = property on="Select Auto" class="CmbBox"("Strings[]"=w641) -> ()  [unwired: 2 in, 2 out]
      }
      event "Select Auto": Value Change {
        # "User modified the Auto Selection. Write to NT variable so robot knows."
        n385 = event-data() -> ("NewVal"=w644:string)  [unwired: 1 in]
        n386 = call <vilib>:"NT Write String.vi"("String"=w644, "Name"="Auto Selector") -> ()  [unwired: 9 in, 1 out]
      }
      event "Command Selection": Value Change {
        # "Get the params and show in table"
        n387 = event-data() -> ("NewVal"=w650:i32)  [unwired: 1 in]
        n388 = property on="Command Selection" class="MCListbox (strict)"() -> ("ItemNames"=w648:string[][])  [unwired: 2 in, 2 out]
        n389 = call <vilib>:"WPI_DashboardUpdate Command Params.vi"("NewVal"=w650, "Commands"=w648, "Param Tbl"=w649) -> ()  [unwired: 8 in, 1 out]
      }
      event "Execute Command": Value Change {
        # "Started one, Unique ID holds\nresponse"
        n390 = event-data() -> ()  [unwired: 1 in, 1 out]
        n391 = property on="Command Selection" class="MCListbox (strict)"() -> ("ItemNames"=w661:string[][])  [unwired: 2 in, 2 out]
        n392 = Index Array(array=w661, index (row)="Command Selection", index (col)=0) -> (element=w659:string)
        n393 = call <vilib>:"Invoke Commands.vi"("Command Params"="Command Params", "Function Name"=w659) -> ("Params"=w655:u8, "Started"=w654:bool)  [unwired: 7 in, 1 out]
        n394 = Array Subset(array="Command Params", length (row)=w655) -> (w656:string[][])  [unwired: 3 in]
        n395 = Select(t="Executing" ("Cmd Status"), s=w654, f="" ("Cmd Status")) -> (s? t:f=→"Cmd Status":string)
      }
      event "Command Selection": Double Click {
        n396 = event-data() -> ("Row"=w669:i32)  [unwired: 1 in]
        n397 = property on="Command Selection" class="MCListbox (strict)"() -> ("ItemNames"=w672:string[][])  [unwired: 2 in, 2 out]
        n398 = local read "Command Params"() -> (w668:string[][])
        n399 = Index Array(array=w672, index (row)=w669, index (col)=0) -> (element=w670:string)
        n400 = call <vilib>:"Invoke Commands.vi"("Command Params"=w668, "Function Name"=w670) -> ("Params"=w667:u8, "Started"=w662:bool)  [unwired: 7 in, 1 out]
        n401 = Array Subset(array=w668, length (row)=w667) -> (w666:string[][])  [unwired: 3 in]
        n402 = Select(t="Executing" ("Cmd Status"), s=w662, f="" ("Cmd Status")) -> (s? t:f=w663:string)
        n403 = local write "Cmd Status"(w663) -> ()
      }
      event "CheckList": Double Click {
        # "Shift clears all"
        # "Update symbols on the listbox"
        n404 = event-data() -> ("PlatMods.Shift"=w674:bool, "Row"=w676:i32)  [unwired: 1 in]
        n405 = case shown="True" w674 {
          tunnel: w676 -> [w680 _]
          tunnel: 1 -> [w679 _]
          frame False {
            n406 = property on="CheckList" class="LstBox (strict)"() -> ("Item Symbols"=w678:i32[])  [unwired: 2 in, 2 out]
            n407 = Replace Array Subset(array=w678, new element=w679, index=w680) -> (w677:i32[])
            n408 = property on="CheckList" class="LstBox (strict)"("Item Symbols"=w677) -> ()  [unwired: 2 in, 2 out]
          }
          frame True {
            w681 = 0 ("Top Row")
            n409 = property on="CheckList" class="LstBox (strict)"() -> ("Number of Rows"=w683:u32)  [unwired: 2 in, 2 out]
            n410 = Initialize Array(0, w683) -> (w682:i32[])
            n411 = property on="CheckList" class="LstBox (strict)"("Top Row"=w681, "Value"=w681, "Item Symbols"=w682) -> ()  [unwired: 2 in, 2 out]
          }
        }
      }
      event "CheckList": Key Down {
        # "Update symbols on the listbox\nLeft and right keys check and uncheck"
        n412 = event-data() -> ("VKey"=w687:T27)  [unwired: 1 in]
        n413 = case shown="\"Left\", \"Right\"" w687 {
          selector: w687 -> [w692 _]
          tunnel: eventvkey."Left" ("VKey") -> [w690 _]
          frame "Left", "Right" {
            n414 = Equal?(x=w690, y=w692) -> (x = y?=w691:bool)
            n415 = Select(t=0, s=w691, f=1) -> (s? t:f=w693:i32)
            n416 = property on="CheckList" class="LstBox (strict)"() -> ("Item Symbols"=w696:i32[])  [unwired: 2 in, 2 out]
            n417 = Replace Array Subset(array=w696, new element=w693, index="CheckList") -> (w695:i32[])
            n418 = property on="CheckList" class="LstBox (strict)"("Item Symbols"=w695) -> ()  [unwired: 2 in, 2 out]
          }
          frame Default {
          }
        }
      }
      event "Motor.Enable": Value Change {
        # "When the test mode otor enable helper is set, update that\ntree row item's value"
        n419 = event-data() -> ("NewVal"=w702:bool)  [unwired: 1 in]
        n420 = Unbundle("Motor") -> ("Value"=w701:dbl)  [unwired: 1 out]
        n421 = Select(t=w701, s=w702, f=0.0) -> (s? t:f=w699:dbl)
        n422 = call <vilib>:"NT Write Number.vi"("Numeric"=w699, "Name"=w698) -> ()  [unwired: 9 in, 1 out]
      }
      event "Test Slider": Value Change {
        # "When the test mode slider helper is set, update that\ntree row item's value"
        n423 = event-data() -> ("NewVal"=w705:dbl)  [unwired: 1 in]
        n424 = call <vilib>:"NT Write Number.vi"("Numeric"=w705, "Name"=w706) -> ()  [unwired: 9 in, 1 out]
      }
      event "On/Off": Value Change {
        # "When the test mode on/off helper value is set, update that\ntree row item's value"
        n425 = event-data() -> ("NewVal"=w710:bool)  [unwired: 1 in]
        n426 = Boolean To (0,1)(Boolean=w710) -> (0, 1=w709:i16)
        n427 = call <vilib>:"NT Write Number.vi"("Numeric"=w709, "Name"=w708) -> ()  [unwired: 9 in, 1 out]
      }
      event "Rev/Fwd": Value Change {
        # "When the test mode helper value for relays is set, update that\ntree row item's value"
        n428 = event-data() -> ("NewVal.Forward"=w718:bool, "NewVal.Reverse"=w717:bool)  [unwired: 1 in]
        n429 = Boolean To (0,1)(Boolean=w718) -> (0, 1=w714:i16)
        n430 = Boolean To (0,1)(Boolean=w717) -> (0, 1=w716:i16)
        n431 = Negate(x=w716) -> (-x=w715:i16)
        n432 = Add(x=w714, y=w715) -> (x+y=w713:i16)
        n433 = call <vilib>:"NT Write Number.vi"("Numeric"=w713, "Name"=w712) -> ()  [unwired: 9 in, 1 out]
      }
      event "Test Ring": Value Change {
        # "When a test mode helper value is selected from the ring,\nset the tree item's variable to the string value"
        n434 = event-data() -> ("NewVal"=w722:u16)  [unwired: 1 in]
        n435 = property on="Test Ring" class="Ring (strict)"() -> ("Strings []"=w723:string[])  [unwired: 2 in, 2 out]
        n436 = Index Array(array=w723, index=w722) -> (element=w721:string)
        n437 = call <vilib>:"NT Write String.vi"("String"=w721, "Name"=w720) -> ()  [unwired: 9 in, 1 out]
      }
      event "Rec Mode": Value Change {
        # "Update globals for recording mode and path to read log from.\nClear when logging and let NetworkTables set path for vision to\nuse."
        n438 = event-data() -> ("NewVal"=w734:enum32{"Stop", "Record", "Playback"})  [unwired: 1 in]
        n439 = global write "WPI_DashboardLogging Global.vi" "Logging Filename"(path "") -> ()
        n440 = global write "WPI_DashboardLogging Global.vi" "Recording"(w734) -> ()
        n441 = case shown="\"Playback\"" w734 {
          tunnel: w733 -> [_ w736 w745]
          tunnel: [_ _ w744] -> w731
          tunnel: [_ _ w743] -> _
          tunnel: w729 -> [_ _ w741]
          tunnel: cluster{i32, i32} {-250, 170} -> [_ _ w740]
          tunnel: [_ _ T28 {"Image Size"=TRUE, "Image Type"=TRUE, "Pixel Value"=TRUE, "ROI Information"=TRUE, "Zoom Factor"=FALSE} ("Image Information Shown:All Elements")] -> w724
          tunnel: [_ _ TRUE ("Zoom Factor")] -> w725
          tunnel: w727 -> [_ _ w737]
          frame Default {
          }
          frame "Stop", "Record" {
            # "Place Window too"
            n442 = invoke class="VI" method="FP.Close"(reference=w736) -> (reference out=w735:refnum<vi>)  [unwired: 2 in, 2 out]
            n443 = invoke class="VI" method="Abort VI"(reference=w735) -> ()  [unwired: 2 in, 3 out]
          }
          frame "Playback" {
            n444 = call "Open Playback Panel.vi"("Offset"=w740, "DB VI Ref"=w741, "Playback in"=w745) -> ("Playback out"=w742:refnum<vi>)  [unwired: 8 in]
            n445 = register-events(w742, w737) -> (reference out=w744:refnum<event-registration>, error out=w743:errorcluster)  [unwired: 2 in]
          }
        }
        n446 = property on="Camera Image Right" class="ImageControl"("Image Information Shown"=w724, "Image Information Visible"=w725) -> ()  [unwired: 2 in, 2 out]
        n447 = property on="Camera Image" class="ImageControl"("Image Information Shown"=w724, "Image Information Visible"=w725) -> ()  [unwired: 2 in, 2 out]
        n448 = call <vilib>:"WPI_DashboardNT Log FieldName Cache.vi"("Operation"=enum16{"Lookup/Add", "Index", "Clear"}."Clear") -> ()  [unwired: 8 in, 3 out]
      }
      event Panel Close {
        w747 = enum32{"Stop", "Record", "Playback"}."Stop" ("Rec Mode")
        # "Playback window has been closed, abort"
        n449 = event-data() -> ()  [unwired: 1 in, 4 out]
        n450 = local write "Rec Mode"(w747) -> ()
        n451 = global write "WPI_DashboardLogging Global.vi" "Recording"(w747) -> ()
      }
      event Panel Close {
        # "Abort playback window and ourself"
        n452 = event-data() -> ()  [unwired: 1 in, 4 out]
        n453 = invoke class="VI" method="FP.Close"(reference=w751) -> (reference out=w750:refnum<vi>)  [unwired: 2 in, 2 out]
        n454 = invoke class="VI" method="Abort VI"(reference=w750) -> (error out=w749:errorcluster)  [unwired: 2 in, 2 out]
        n455 = invoke class="VI" method="Abort VI"(error in=w749) -> ()  [unwired: 2 in, 3 out]
      }
      event User Event {
        n456 = event-data() -> ("IDs"=w758:cluster{"RPC field ID":u16, "Unique ID":u16}, "String"=w757:string)  [unwired: 1 in]
        n457 = Bundle("IDs"=w758, "String"=w757) -> (w756:T12)  [unwired: 1 in]
        n458 = call <vilib>:"Retrieve RPC Response.vi"("RPC Response"=w756) -> ("Output"=w754:string[][])  [unwired: 10 in]
        n459 = Build Array (concatenate)(w752, w754) -> (w753:string[][])
        n460 = local write "Command Params"(w753) -> ()
        n461 = local write "Cmd Status"("" ("Cmd Status")) -> ()
      }
      event "Tree": Double Click {
        n462 = event-data() -> ("PlatMods"=w764:T31, "Tag"=w761:string)  [unwired: 1 in]
        n463 = Unbundle(w764) -> ("Shift"=w763:bool)  [unwired: 4 out]
        n464 = String Subset(string=w761, length (rest)=1 ("length (rest)")) -> (substring=w760:string)  [unwired: 1 in]
        n465 = Not(x=w763) -> (.not. x?=w762:bool)
        n466 = case shown="\"/\"" w760 {
          tunnel: w761 -> [_ w767]
          tunnel: w762 -> [_ w766]
          frame Default {
          }
          frame "/" {
            n467 = call <vilib>:"NT Update Persistence.vi"("Persistence"=w766, "Name"=w767) -> ()  [unwired: 9 in, 1 out]
          }
        }
      }
    }
  }
  n468 = while {
    tunnel: w66 -> [w769]
    i -> [w772]
    stop <- FALSE stop-if-true
    n469 = Wait (ms)(milliseconds to wait=u32 100) -> ()  [unwired: 1 out]
    n470 = case shown="\"Playback\"" "Rec Mode" {
      tunnel: w772 -> [_ _ w787]
      tunnel: [u32 2829099 ("Base Color") u32 11141120 ("Target Color") w776] -> w768
      frame "Stop", Default {
        # "Reset the color, extra updates don't cost much"
      }
      frame "Record" {
      }
      frame "Playback" {
        # "Playback"
        n471 = Quotient & Remainder(x=w787, y=u32 50 ("milliseconds to wait")) -> (x-y*floor(x/y)=w783:u32)  [unwired: 1 out]
        n472 = Divide(x=w783, y=u32 50 ("milliseconds to wait")) -> (x/y=w780:dbl)
        n473 = Multiply(x=6.283185307179586, y=w780) -> (x*y=w785:dbl)
        n474 = Sine(x=w785) -> (sin(x)=w784:dbl)
        n475 = Absolute Value(x=w784) -> (abs(x)=w777:dbl)
        n476 = call "Interpolate RGB Color.vi"("Proportion"=w777, "Target Color"=u32 30976, "Base Color"=u32 2829099) -> ("Result Color"=w776:u32)  [unwired: 8 in]
      }
    }
    n477 = property class="Pane"(reference=w769, "PaneColor"=w768) -> ()  [unwired: 1 in, 2 out]
  }
  n478 = local write "Dashboard Tab"(T2."Drive" ("Dashboard Tab")) -> ()
  n479 = property on="On/Off" class="Bool (strict)"("Visible"=w37) -> ()  [unwired: 2 in, 2 out]
  n480 = property on="Motor" class="Clust (strict)"("Visible"=w37) -> ()  [unwired: 2 in, 2 out]
  n481 = property on="Progress" class="Clust (strict)"("Visible"=w37) -> ()  [unwired: 2 in, 2 out]
  n482 = property on="Test Ring" class="Ring (strict)"("Visible"=w37) -> ()  [unwired: 2 in, 2 out]
  n483 = property on="Rev/Fwd" class="Clust (strict)"("Visible"=w37) -> ()  [unwired: 2 in, 2 out]
  n484 = while {
    tunnel: u16 1741 ("timeout ms (25000)") -> [w789]
    stop <- FALSE stop-if-true
    n485 = TCP Create Listener(10:w789) -> (0:w788:errorcluster, 3:w790:refnum<k5>)  [unwired: 4 in, 1 out]
    n486 = case shown="No Error" w788 {
      selector: w788 -> [w792 _]
      tunnel: w790 -> [w793 _]
      frame No Error {
        n487 = while {
          tunnel: w793 -> [w796]
          tunnel: w792 -> [w795]
          stop <- FALSE stop-if-true
          n488 = TCP Wait On Listener(8:w795, 11:w796) -> (0:w797:errorcluster, 4:w798:refnum<k5>)  [unwired: 2 in, 3 out]
          n489 = local write "TCP"(w798) -> ()
          n490 = case shown="No Error" w797 {
            frame No Error {
            }
            frame Error {
              n491 = Wait (ms)(milliseconds to wait=u32 1000) -> ()  [unwired: 1 out]
            }
          }
        }
      }
      frame Error {
        n492 = Wait (ms)(milliseconds to wait=u32 1000) -> ()  [unwired: 1 out]
      }
    }
  }
  n493 = local write "Command Selection"(u16 0 ("milliseconds to wait")) -> ()
  n494 = local write "Command Params"(string[][] [] ("Command Params")) -> ()
  n495 = global write "WPI_DashboardLogging Global.vi" "Recording"(w60) -> ()
  n496 = local write "Rec Mode"(w60) -> ()
  n497 = call <vilib>:"NT Write String.vi"("String"="Select Auto", "Name"="Auto Selector") -> ()  [unwired: 9 in, 1 out]
